vi "Scan Control Data Element.vi"(7 "Body":string, 8 "error in (no error)":errorcluster, 11 "Type/Default in":variant) -> (0 "error out":errorcluster, 3 "Type/Default out":variant)   [LabVIEW 2023, in "Request.lvclass"]
uses:
  Request.lvclass
  <vilib>/Utility/Data Type/NI_Data Type.lvlib
  <vilib>/wsapi/NI_WebServices.lvlib
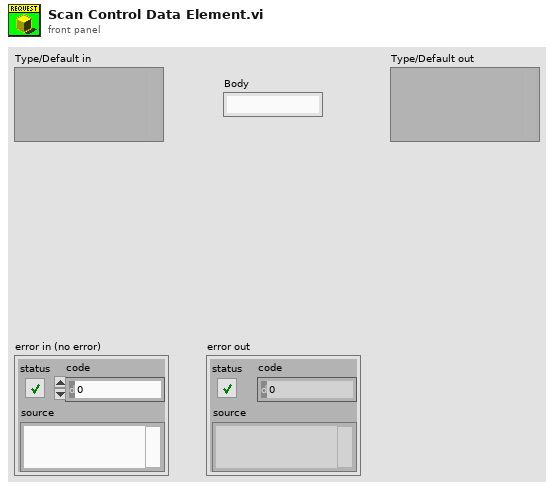
[diagram p1: front panel]
types:
  T1 = typedef "NI_Data Type.lvlib/Data Type.ctl" = enum8{"Invalid Type", "Void", "I8", "I16", "I32", "I64", "U8", "U16", "U32", "U64", "Single Float", "Double Float", "Extended Float", "Single Complex", "Double Complex", "Extended Complex", "Enum U8", "Enum U16", "Enum U32", "Enum U64", "Single Float With Unit", "Double Float With Unit", "Extended Float With Unit", "Single Complex with Unit", "Double Complex with Unit", "Extended Complex with Unit", "Boolean", "String", "Path", "Picture", "Tag", "Array", "Cluster", "Variant", "LV Variant", "Waveform", "Timestamp", "Digital Waveform", "Digital Data", "ExpressData", "Refnum", "External Data", "VI", "Poly VI", "LabVIEW Class Instance", "Fixed Point", "Set Collection", "Map Collection"}
  T2 = typedef "imagedata.ctl" = cluster{"image type":i32, "image depth":i32, "image":u8[], "mask":u8[], "colors":u32[], "Rectangle":cluster{"left":i16, "top":i16, "right":i16, "bottom":i16}}
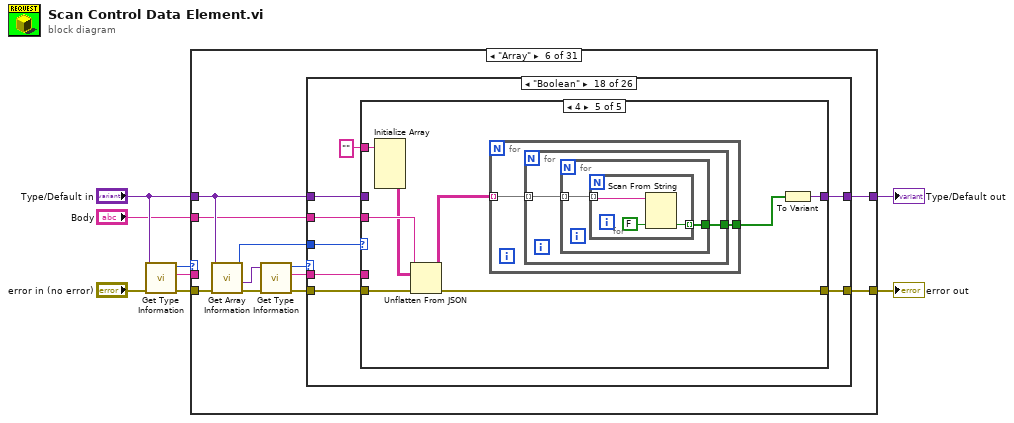
[diagram p0: block diagram]
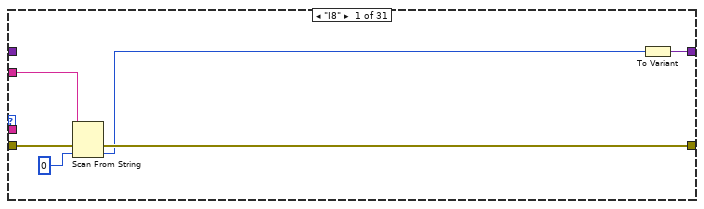
[diagram p2: hidden frame]
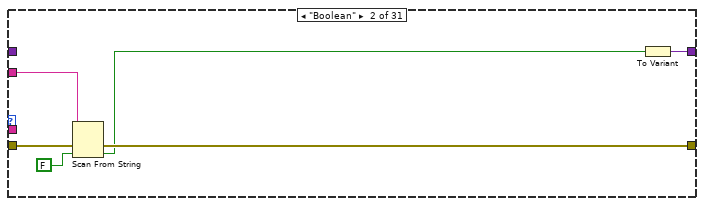
[diagram p3: hidden frame]
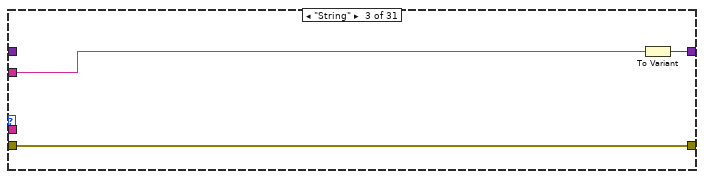
[diagram p4: hidden frame]
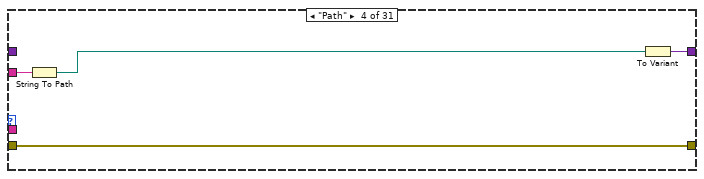
[diagram p5: hidden frame]
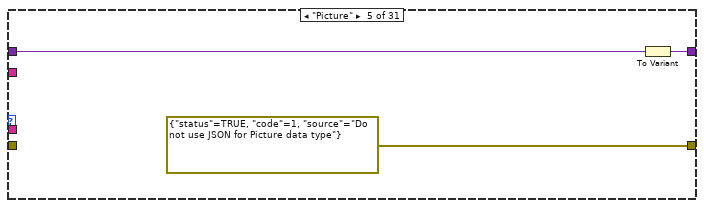
[diagram p6: hidden frame]
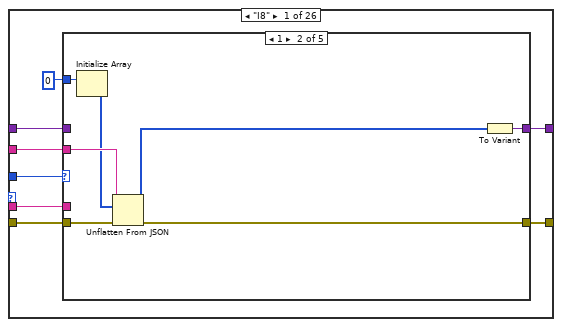
[diagram p7: hidden frame]
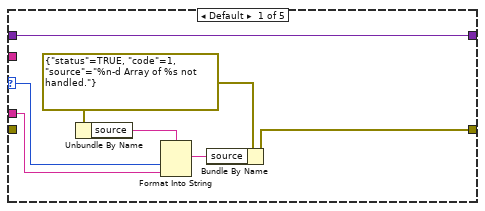
[diagram p8: hidden frame]
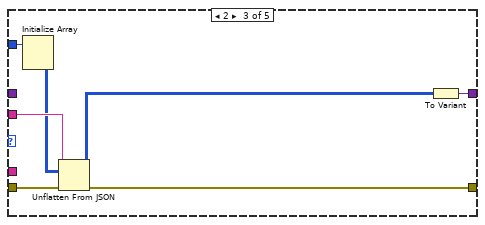
[diagram p9: hidden frame]
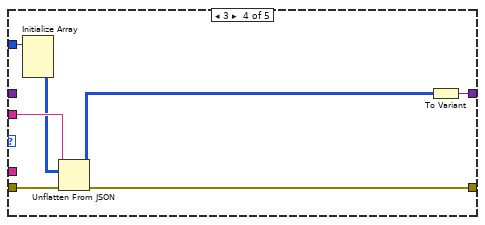
[diagram p10: hidden frame]
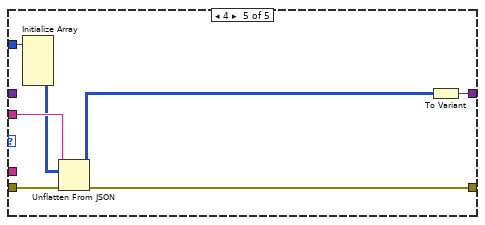
[diagram p11: hidden frame]
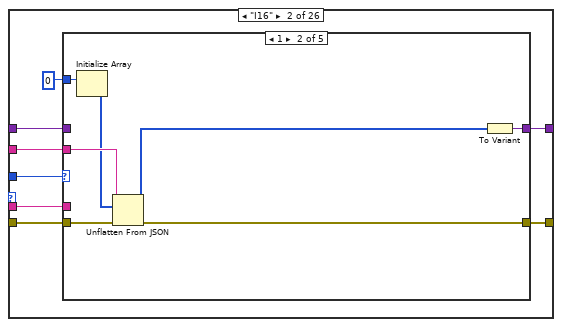
[diagram p12: hidden frame]
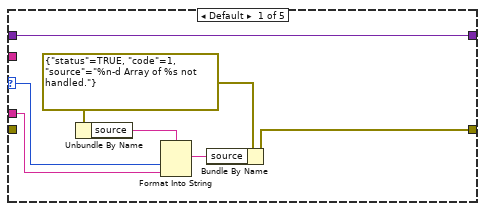
[diagram p13: hidden frame]
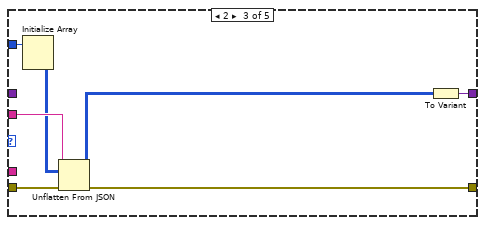
[diagram p14: hidden frame]
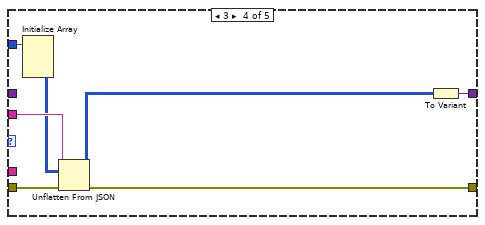
[diagram p15: hidden frame]
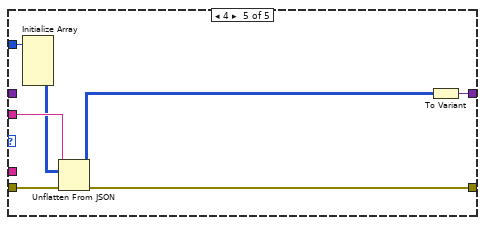
[diagram p16: hidden frame]
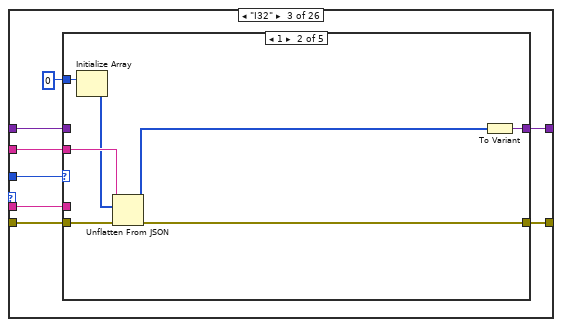
[diagram p17: hidden frame]
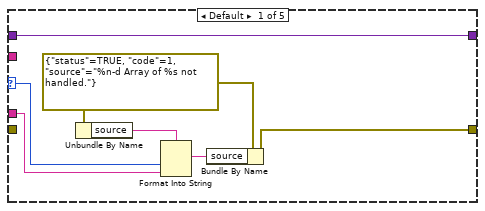
[diagram p18: hidden frame]
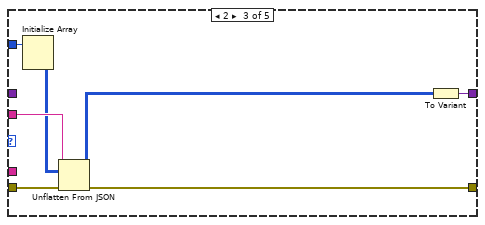
[diagram p19: hidden frame]
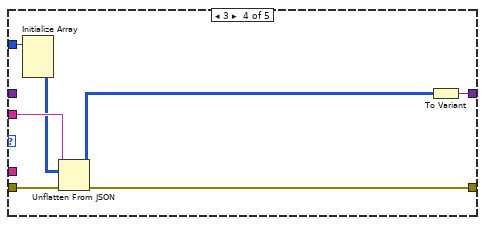
[diagram p20: hidden frame]
diagram:
  n1 = call <vilib>:"Get Type Information.vi"("error in (no error)"="error in (no error)", "variant"="Type/Default in") -> ("error out"=w7:errorcluster, "name"=w8:string, "type"=w3:T1)  [unwired: 5 in, 2 out]
  n2 = case shown="\"Array\"" w3 {
    tunnel: [w10 w16 w23 w27 w30 w41 w1308 w1330 w1336 w1342 w1348 w1354 w1360 w1366 w1372 w1378 w1384 w1390 w1396 w1402 w1408 w1414 w1420 w1426 w1432 w1438 w1450 w1458 w1466 w1474 w1480] -> w4
    tunnel: "Type/Default in" -> [_ _ _ _ w28 w39 w1308 _ _ _ _ _ _ _ _ _ _ _ _ _ _ _ _ _ _ _ w1449 w1457 w1465 w1473 w1480]
    tunnel: [w13 w19 w21 w25 errorcluster {"status"=TRUE, "code"=1, "source"="Do not use JSON for Picture data type"} ("error out") w33 w1309 w1333 w1339 w1345 w1351 w1357 w1363 w1369 w1375 w1381 w1387 w1393 w1399 w1405 w1411 w1417 w1423 w1429 w1435 w1441 w1444 w1452 w1460 w1468 w1475] -> w6
    tunnel: w7 -> [w14 w20 w21 w25 _ w40 w1312 w1334 w1340 w1346 w1352 w1358 w1364 w1370 w1376 w1382 w1388 w1394 w1400 w1406 w1412 w1418 w1424 w1430 w1436 w1442 w1448 w1456 w1464 w1472 _]
    tunnel: "Body" -> [w12 w18 w22 w26 _ w32 w1307 w1332 w1338 w1344 w1350 w1356 w1362 w1368 w1374 w1380 w1386 w1392 w1398 w1404 w1410 w1416 w1422 w1428 w1434 w1440 w1446 w1454 w1462 w1470 _]
    tunnel: w8 -> [_ _ _ _ _ _ _ _ _ _ _ _ _ _ _ _ _ _ _ _ _ _ _ _ _ _ _ _ _ _ w1477]
    frame "I8" {
      n3 = Scan From String(input string=w12, error in=w14, default 1=i8 0 ("default value 1")) -> (error out=w13:errorcluster, output 1=w9:i8)  [unwired: 2 in, 2 out]
      n4 = To Variant(anything=w9) -> (Variant=w10:variant)
    }
    frame "Boolean" {
      n5 = Scan From String(input string=w18, error in=w20, default 1=FALSE) -> (error out=w19:errorcluster, output 1=w15:bool)  [unwired: 2 in, 2 out]
      n6 = To Variant(anything=w15) -> (Variant=w16:variant)
    }
    frame "String" {
      n7 = To Variant(anything=w22) -> (Variant=w23:variant)
    }
    frame "Path" {
      n8 = String To Path(string=w26) -> (path=w24:path)
      n9 = To Variant(anything=w24) -> (Variant=w27:variant)
    }
    frame "Picture" {
      n10 = To Variant(anything=w28) -> (Variant=w30:variant)
    }
    frame "Array" {
      n11 = call <vilib>:"Get Array Information.vi"("error in (no error)"=w40, "variant"=w39) -> ("error out"=w38:errorcluster, "array element data type"=w37:variant, "number of dimensions"=w31:i32)  [unwired: 6 in, 1 out]
      n12 = call <vilib>:"Get Type Information.vi"("error in (no error)"=w38, "variant"=w37) -> ("error out"=w36:errorcluster, "name"=w34:string, "type"=w35:T1)  [unwired: 5 in, 2 out]
      n13 = case shown="\"Boolean\"" w35 {
        tunnel: [w45 w88 w131 w174 w217 w260 w303 w346 w389 w432 w475 w518 w561 w604 w647 w690 w733 w776 w847 w890 w937 w1028 w1097 w1166 w1235 w1301] -> w41
        tunnel: w39 -> [w43 w86 w129 w172 w215 w258 w301 w344 w387 w430 w473 w516 w559 w602 w645 w688 w731 w774 w845 w888 w935 w1026 w1095 w1164 w1233 w1301]
        tunnel: w36 -> [w47 w90 w133 w176 w219 w262 w305 w348 w391 w434 w477 w520 w563 w606 w649 w692 w735 w778 w849 w892 w939 w1030 w1099 w1168 w1237 _]
        tunnel: w34 -> [w42 w85 w128 w171 w214 w257 w300 w343 w386 w429 w472 w515 w558 w601 w644 w687 w730 w773 w844 w887 w934 w1025 w1094 w1163 w1232 w1303]
        tunnel: [w44 w87 w130 w173 w216 w259 w302 w345 w388 w431 w474 w517 w560 w603 w646 w689 w732 w775 w846 w889 w936 w1027 w1096 w1165 w1234 w1302] -> w33
        tunnel: w32 -> [w46 w89 w132 w175 w218 w261 w304 w347 w390 w433 w476 w519 w562 w605 w648 w691 w734 w777 w848 w891 w938 w1029 w1098 w1167 w1236 _]
        tunnel: w31 -> [w49 w92 w135 w178 w221 w264 w307 w350 w393 w436 w479 w522 w565 w608 w651 w694 w737 w780 w851 w894 w941 w1032 w1101 w1170 w1239 _]
        frame "I8" {
          n14 = case shown="1" w49 {
            selector: w49 -> [w52 _ _ _ _]
            tunnel: i8 0 -> [_ w63 w70 w77 w84]
            tunnel: w47 -> [_ w62 w69 w76 w83]
            tunnel: w46 -> [_ w61 w68 w75 w82]
            tunnel: [w56 w58 w65 w72 w79] -> w45
            tunnel: [w50 w57 w64 w71 w78] -> w44
            tunnel: w43 -> [w56 _ _ _ _]
            tunnel: w42 -> [w51 _ _ _ _]
            frame Default {
              w53 = errorcluster {"status"=TRUE, "code"=1, "source"="%n-d Array of %s not handled."} ("error out")
              n15 = Unbundle By Name(w53) -> ("source"=w54:string)
              n16 = Format Into String(format string=w54, w52, w51) -> (resulting string=w55:string)  [unwired: 2 in, 1 out]
              n17 = Bundle By Name(cluster=w53, "source"=w55) -> (w50:errorcluster)
            }
            frame 1 {
              n18 = Initialize Array(w63) -> (w60:i8[])  [unwired: 1 in]
              n19 = Unflatten From JSON(JSON string=w61, type and defaults=w60, error in (no error)=w62) -> (value=w59:i8[], error out=w57:errorcluster)  [unwired: 4 in]
              n20 = To Variant(anything=w59) -> (Variant=w58:variant)
            }
            frame 2 {
              n21 = Initialize Array(w70) -> (w67:i8[][])  [unwired: 2 in]
              n22 = Unflatten From JSON(JSON string=w68, type and defaults=w67, error in (no error)=w69) -> (value=w66:i8[][], error out=w64:errorcluster)  [unwired: 4 in]
              n23 = To Variant(anything=w66) -> (Variant=w65:variant)
            }
            frame 3 {
              n24 = Initialize Array(w77) -> (w74:i8[][][])  [unwired: 3 in]
              n25 = Unflatten From JSON(JSON string=w75, type and defaults=w74, error in (no error)=w76) -> (value=w73:i8[][][], error out=w71:errorcluster)  [unwired: 4 in]
              n26 = To Variant(anything=w73) -> (Variant=w72:variant)
            }
            frame 4 {
              n27 = Initialize Array(w84) -> (w81:i8[][][][])  [unwired: 4 in]
              n28 = Unflatten From JSON(JSON string=w82, type and defaults=w81, error in (no error)=w83) -> (value=w80:i8[][][][], error out=w78:errorcluster)  [unwired: 4 in]
              n29 = To Variant(anything=w80) -> (Variant=w79:variant)
            }
          }
        }
        frame "I16" {
          n30 = case shown="1" w92 {
            selector: w92 -> [w95 _ _ _ _]
            tunnel: i16 0 -> [_ w106 w113 w120 w127]
            tunnel: w90 -> [_ w105 w112 w119 w126]
            tunnel: w89 -> [_ w104 w111 w118 w125]
            tunnel: [w99 w101 w108 w115 w122] -> w88
            tunnel: [w93 w100 w107 w114 w121] -> w87
            tunnel: w86 -> [w99 _ _ _ _]
            tunnel: w85 -> [w94 _ _ _ _]
            frame Default {
              w96 = errorcluster {"status"=TRUE, "code"=1, "source"="%n-d Array of %s not handled."} ("error out")
              n31 = Unbundle By Name(w96) -> ("source"=w97:string)
              n32 = Format Into String(format string=w97, w95, w94) -> (resulting string=w98:string)  [unwired: 2 in, 1 out]
              n33 = Bundle By Name(cluster=w96, "source"=w98) -> (w93:errorcluster)
            }
            frame 1 {
              n34 = Initialize Array(w106) -> (w103:i16[])  [unwired: 1 in]
              n35 = Unflatten From JSON(JSON string=w104, type and defaults=w103, error in (no error)=w105) -> (value=w102:i16[], error out=w100:errorcluster)  [unwired: 4 in]
              n36 = To Variant(anything=w102) -> (Variant=w101:variant)
            }
            frame 2 {
              n37 = Initialize Array(w113) -> (w110:i16[][])  [unwired: 2 in]
              n38 = Unflatten From JSON(JSON string=w111, type and defaults=w110, error in (no error)=w112) -> (value=w109:i16[][], error out=w107:errorcluster)  [unwired: 4 in]
              n39 = To Variant(anything=w109) -> (Variant=w108:variant)
            }
            frame 3 {
              n40 = Initialize Array(w120) -> (w117:i16[][][])  [unwired: 3 in]
              n41 = Unflatten From JSON(JSON string=w118, type and defaults=w117, error in (no error)=w119) -> (value=w116:i16[][][], error out=w114:errorcluster)  [unwired: 4 in]
              n42 = To Variant(anything=w116) -> (Variant=w115:variant)
            }
            frame 4 {
              n43 = Initialize Array(w127) -> (w124:i16[][][][])  [unwired: 4 in]
              n44 = Unflatten From JSON(JSON string=w125, type and defaults=w124, error in (no error)=w126) -> (value=w123:i16[][][][], error out=w121:errorcluster)  [unwired: 4 in]
              n45 = To Variant(anything=w123) -> (Variant=w122:variant)
            }
          }
        }
        frame "I32" {
          n46 = case shown="1" w135 {
            selector: w135 -> [w138 _ _ _ _]
            tunnel: 0 -> [_ w149 w156 w163 w170]
            tunnel: w133 -> [_ w148 w155 w162 w169]
            tunnel: w132 -> [_ w147 w154 w161 w168]
            tunnel: [w142 w144 w151 w158 w165] -> w131
            tunnel: [w136 w143 w150 w157 w164] -> w130
            tunnel: w129 -> [w142 _ _ _ _]
            tunnel: w128 -> [w137 _ _ _ _]
            frame Default {
              w139 = errorcluster {"status"=TRUE, "code"=1, "source"="%n-d Array of %s not handled."} ("error out")
              n47 = Unbundle By Name(w139) -> ("source"=w140:string)
              n48 = Format Into String(format string=w140, w138, w137) -> (resulting string=w141:string)  [unwired: 2 in, 1 out]
              n49 = Bundle By Name(cluster=w139, "source"=w141) -> (w136:errorcluster)
            }
            frame 1 {
              n50 = Initialize Array(w149) -> (w146:i32[])  [unwired: 1 in]
              n51 = Unflatten From JSON(JSON string=w147, type and defaults=w146, error in (no error)=w148) -> (value=w145:i32[], error out=w143:errorcluster)  [unwired: 4 in]
              n52 = To Variant(anything=w145) -> (Variant=w144:variant)
            }
            frame 2 {
              n53 = Initialize Array(w156) -> (w153:i32[][])  [unwired: 2 in]
              n54 = Unflatten From JSON(JSON string=w154, type and defaults=w153, error in (no error)=w155) -> (value=w152:i32[][], error out=w150:errorcluster)  [unwired: 4 in]
              n55 = To Variant(anything=w152) -> (Variant=w151:variant)
            }
            frame 3 {
              n56 = Initialize Array(w163) -> (w160:i32[][][])  [unwired: 3 in]
              n57 = Unflatten From JSON(JSON string=w161, type and defaults=w160, error in (no error)=w162) -> (value=w159:i32[][][], error out=w157:errorcluster)  [unwired: 4 in]
              n58 = To Variant(anything=w159) -> (Variant=w158:variant)
            }
            frame 4 {
              n59 = Initialize Array(w170) -> (w167:i32[][][][])  [unwired: 4 in]
              n60 = Unflatten From JSON(JSON string=w168, type and defaults=w167, error in (no error)=w169) -> (value=w166:i32[][][][], error out=w164:errorcluster)  [unwired: 4 in]
              n61 = To Variant(anything=w166) -> (Variant=w165:variant)
            }
          }
        }
        frame "I64" {
          n62 = case shown="1" w178 {
            selector: w178 -> [w181 _ _ _ _]
            tunnel: i64 0 -> [_ w192 w199 w206 w213]
            tunnel: w176 -> [_ w191 w198 w205 w212]
            tunnel: w175 -> [_ w190 w197 w204 w211]
            tunnel: [w185 w187 w194 w201 w208] -> w174
            tunnel: [w179 w186 w193 w200 w207] -> w173
            tunnel: w172 -> [w185 _ _ _ _]
            tunnel: w171 -> [w180 _ _ _ _]
            frame Default {
              w182 = errorcluster {"status"=TRUE, "code"=1, "source"="%n-d Array of %s not handled."} ("error out")
              n63 = Unbundle By Name(w182) -> ("source"=w183:string)
              n64 = Format Into String(format string=w183, w181, w180) -> (resulting string=w184:string)  [unwired: 2 in, 1 out]
              n65 = Bundle By Name(cluster=w182, "source"=w184) -> (w179:errorcluster)
            }
            frame 1 {
              n66 = Initialize Array(w192) -> (w189:i64[])  [unwired: 1 in]
              n67 = Unflatten From JSON(JSON string=w190, type and defaults=w189, error in (no error)=w191) -> (value=w188:i64[], error out=w186:errorcluster)  [unwired: 4 in]
              n68 = To Variant(anything=w188) -> (Variant=w187:variant)
            }
            frame 2 {
              n69 = Initialize Array(w199) -> (w196:i64[][])  [unwired: 2 in]
              n70 = Unflatten From JSON(JSON string=w197, type and defaults=w196, error in (no error)=w198) -> (value=w195:i64[][], error out=w193:errorcluster)  [unwired: 4 in]
              n71 = To Variant(anything=w195) -> (Variant=w194:variant)
            }
            frame 3 {
              n72 = Initialize Array(w206) -> (w203:i64[][][])  [unwired: 3 in]
              n73 = Unflatten From JSON(JSON string=w204, type and defaults=w203, error in (no error)=w205) -> (value=w202:i64[][][], error out=w200:errorcluster)  [unwired: 4 in]
              n74 = To Variant(anything=w202) -> (Variant=w201:variant)
            }
            frame 4 {
              n75 = Initialize Array(w213) -> (w210:i64[][][][])  [unwired: 4 in]
              n76 = Unflatten From JSON(JSON string=w211, type and defaults=w210, error in (no error)=w212) -> (value=w209:i64[][][][], error out=w207:errorcluster)  [unwired: 4 in]
              n77 = To Variant(anything=w209) -> (Variant=w208:variant)
            }
          }
        }
        frame "U8" {
          n78 = case shown="1" w221 {
            selector: w221 -> [w224 _ _ _ _]
            tunnel: u8 0 -> [_ w235 w242 w249 w256]
            tunnel: w219 -> [_ w234 w241 w248 w255]
            tunnel: w218 -> [_ w233 w240 w247 w254]
            tunnel: [w228 w230 w237 w244 w251] -> w217
            tunnel: [w222 w229 w236 w243 w250] -> w216
            tunnel: w215 -> [w228 _ _ _ _]
            tunnel: w214 -> [w223 _ _ _ _]
            frame Default {
              w225 = errorcluster {"status"=TRUE, "code"=1, "source"="%n-d Array of %s not handled."} ("error out")
              n79 = Unbundle By Name(w225) -> ("source"=w226:string)
              n80 = Format Into String(format string=w226, w224, w223) -> (resulting string=w227:string)  [unwired: 2 in, 1 out]
              n81 = Bundle By Name(cluster=w225, "source"=w227) -> (w222:errorcluster)
            }
            frame 1 {
              n82 = Initialize Array(w235) -> (w232:u8[])  [unwired: 1 in]
              n83 = Unflatten From JSON(JSON string=w233, type and defaults=w232, error in (no error)=w234) -> (value=w231:u8[], error out=w229:errorcluster)  [unwired: 4 in]
              n84 = To Variant(anything=w231) -> (Variant=w230:variant)
            }
            frame 2 {
              n85 = Initialize Array(w242) -> (w239:u8[][])  [unwired: 2 in]
              n86 = Unflatten From JSON(JSON string=w240, type and defaults=w239, error in (no error)=w241) -> (value=w238:u8[][], error out=w236:errorcluster)  [unwired: 4 in]
              n87 = To Variant(anything=w238) -> (Variant=w237:variant)
            }
            frame 3 {
              n88 = Initialize Array(w249) -> (w246:u8[][][])  [unwired: 3 in]
              n89 = Unflatten From JSON(JSON string=w247, type and defaults=w246, error in (no error)=w248) -> (value=w245:u8[][][], error out=w243:errorcluster)  [unwired: 4 in]
              n90 = To Variant(anything=w245) -> (Variant=w244:variant)
            }
            frame 4 {
              n91 = Initialize Array(w256) -> (w253:u8[][][][])  [unwired: 4 in]
              n92 = Unflatten From JSON(JSON string=w254, type and defaults=w253, error in (no error)=w255) -> (value=w252:u8[][][][], error out=w250:errorcluster)  [unwired: 4 in]
              n93 = To Variant(anything=w252) -> (Variant=w251:variant)
            }
          }
        }
        frame "U16" {
          n94 = case shown="1" w264 {
            selector: w264 -> [w267 _ _ _ _]
            tunnel: u16 0 -> [_ w278 w285 w292 w299]
            tunnel: w262 -> [_ w277 w284 w291 w298]
            tunnel: w261 -> [_ w276 w283 w290 w297]
            tunnel: [w271 w273 w280 w287 w294] -> w260
            tunnel: [w265 w272 w279 w286 w293] -> w259
            tunnel: w258 -> [w271 _ _ _ _]
            tunnel: w257 -> [w266 _ _ _ _]
            frame Default {
              w268 = errorcluster {"status"=TRUE, "code"=1, "source"="%n-d Array of %s not handled."} ("error out")
              n95 = Unbundle By Name(w268) -> ("source"=w269:string)
              n96 = Format Into String(format string=w269, w267, w266) -> (resulting string=w270:string)  [unwired: 2 in, 1 out]
              n97 = Bundle By Name(cluster=w268, "source"=w270) -> (w265:errorcluster)
            }
            frame 1 {
              n98 = Initialize Array(w278) -> (w275:u16[])  [unwired: 1 in]
              n99 = Unflatten From JSON(JSON string=w276, type and defaults=w275, error in (no error)=w277) -> (value=w274:u16[], error out=w272:errorcluster)  [unwired: 4 in]
              n100 = To Variant(anything=w274) -> (Variant=w273:variant)
            }
            frame 2 {
              n101 = Initialize Array(w285) -> (w282:u16[][])  [unwired: 2 in]
              n102 = Unflatten From JSON(JSON string=w283, type and defaults=w282, error in (no error)=w284) -> (value=w281:u16[][], error out=w279:errorcluster)  [unwired: 4 in]
              n103 = To Variant(anything=w281) -> (Variant=w280:variant)
            }
            frame 3 {
              n104 = Initialize Array(w292) -> (w289:u16[][][])  [unwired: 3 in]
              n105 = Unflatten From JSON(JSON string=w290, type and defaults=w289, error in (no error)=w291) -> (value=w288:u16[][][], error out=w286:errorcluster)  [unwired: 4 in]
              n106 = To Variant(anything=w288) -> (Variant=w287:variant)
            }
            frame 4 {
              n107 = Initialize Array(w299) -> (w296:u16[][][][])  [unwired: 4 in]
              n108 = Unflatten From JSON(JSON string=w297, type and defaults=w296, error in (no error)=w298) -> (value=w295:u16[][][][], error out=w293:errorcluster)  [unwired: 4 in]
              n109 = To Variant(anything=w295) -> (Variant=w294:variant)
            }
          }
        }
        frame "U32" {
          n110 = case shown="1" w307 {
            selector: w307 -> [w310 _ _ _ _]
            tunnel: u32 0 -> [_ w321 w328 w335 w342]
            tunnel: w305 -> [_ w320 w327 w334 w341]
            tunnel: w304 -> [_ w319 w326 w333 w340]
            tunnel: [w314 w316 w323 w330 w337] -> w303
            tunnel: [w308 w315 w322 w329 w336] -> w302
            tunnel: w301 -> [w314 _ _ _ _]
            tunnel: w300 -> [w309 _ _ _ _]
            frame Default {
              w311 = errorcluster {"status"=TRUE, "code"=1, "source"="%n-d Array of %s not handled."} ("error out")
              n111 = Unbundle By Name(w311) -> ("source"=w312:string)
              n112 = Format Into String(format string=w312, w310, w309) -> (resulting string=w313:string)  [unwired: 2 in, 1 out]
              n113 = Bundle By Name(cluster=w311, "source"=w313) -> (w308:errorcluster)
            }
            frame 1 {
              n114 = Initialize Array(w321) -> (w318:u32[])  [unwired: 1 in]
              n115 = Unflatten From JSON(JSON string=w319, type and defaults=w318, error in (no error)=w320) -> (value=w317:u32[], error out=w315:errorcluster)  [unwired: 4 in]
              n116 = To Variant(anything=w317) -> (Variant=w316:variant)
            }
            frame 2 {
              n117 = Initialize Array(w328) -> (w325:u32[][])  [unwired: 2 in]
              n118 = Unflatten From JSON(JSON string=w326, type and defaults=w325, error in (no error)=w327) -> (value=w324:u32[][], error out=w322:errorcluster)  [unwired: 4 in]
              n119 = To Variant(anything=w324) -> (Variant=w323:variant)
            }
            frame 3 {
              n120 = Initialize Array(w335) -> (w332:u32[][][])  [unwired: 3 in]
              n121 = Unflatten From JSON(JSON string=w333, type and defaults=w332, error in (no error)=w334) -> (value=w331:u32[][][], error out=w329:errorcluster)  [unwired: 4 in]
              n122 = To Variant(anything=w331) -> (Variant=w330:variant)
            }
            frame 4 {
              n123 = Initialize Array(w342) -> (w339:u32[][][][])  [unwired: 4 in]
              n124 = Unflatten From JSON(JSON string=w340, type and defaults=w339, error in (no error)=w341) -> (value=w338:u32[][][][], error out=w336:errorcluster)  [unwired: 4 in]
              n125 = To Variant(anything=w338) -> (Variant=w337:variant)
            }
          }
        }
        frame "U64" {
          n126 = case shown="1" w350 {
            selector: w350 -> [w353 _ _ _ _]
            tunnel: u64 0 -> [_ w364 w371 w378 w385]
            tunnel: w348 -> [_ w363 w370 w377 w384]
            tunnel: w347 -> [_ w362 w369 w376 w383]
            tunnel: [w357 w359 w366 w373 w380] -> w346
            tunnel: [w351 w358 w365 w372 w379] -> w345
            tunnel: w344 -> [w357 _ _ _ _]
            tunnel: w343 -> [w352 _ _ _ _]
            frame Default {
              w354 = errorcluster {"status"=TRUE, "code"=1, "source"="%n-d Array of %s not handled."} ("error out")
              n127 = Unbundle By Name(w354) -> ("source"=w355:string)
              n128 = Format Into String(format string=w355, w353, w352) -> (resulting string=w356:string)  [unwired: 2 in, 1 out]
              n129 = Bundle By Name(cluster=w354, "source"=w356) -> (w351:errorcluster)
            }
            frame 1 {
              n130 = Initialize Array(w364) -> (w361:u64[])  [unwired: 1 in]
              n131 = Unflatten From JSON(JSON string=w362, type and defaults=w361, error in (no error)=w363) -> (value=w360:u64[], error out=w358:errorcluster)  [unwired: 4 in]
              n132 = To Variant(anything=w360) -> (Variant=w359:variant)
            }
            frame 2 {
              n133 = Initialize Array(w371) -> (w368:u64[][])  [unwired: 2 in]
              n134 = Unflatten From JSON(JSON string=w369, type and defaults=w368, error in (no error)=w370) -> (value=w367:u64[][], error out=w365:errorcluster)  [unwired: 4 in]
              n135 = To Variant(anything=w367) -> (Variant=w366:variant)
            }
            frame 3 {
              n136 = Initialize Array(w378) -> (w375:u64[][][])  [unwired: 3 in]
              n137 = Unflatten From JSON(JSON string=w376, type and defaults=w375, error in (no error)=w377) -> (value=w374:u64[][][], error out=w372:errorcluster)  [unwired: 4 in]
              n138 = To Variant(anything=w374) -> (Variant=w373:variant)
            }
            frame 4 {
              n139 = Initialize Array(w385) -> (w382:u64[][][][])  [unwired: 4 in]
              n140 = Unflatten From JSON(JSON string=w383, type and defaults=w382, error in (no error)=w384) -> (value=w381:u64[][][][], error out=w379:errorcluster)  [unwired: 4 in]
              n141 = To Variant(anything=w381) -> (Variant=w380:variant)
            }
          }
        }
        frame "Single Float" {
          n142 = case shown="1" w393 {
            selector: w393 -> [w396 _ _ _ _]
            tunnel: sgl 0.0 -> [_ w407 w414 w421 w428]
            tunnel: w391 -> [_ w406 w413 w420 w427]
            tunnel: w390 -> [_ w405 w412 w419 w426]
            tunnel: [w400 w402 w409 w416 w423] -> w389
            tunnel: [w394 w401 w408 w415 w422] -> w388
            tunnel: w387 -> [w400 _ _ _ _]
            tunnel: w386 -> [w395 _ _ _ _]
            frame Default {
              w397 = errorcluster {"status"=TRUE, "code"=1, "source"="%n-d Array of %s not handled."} ("error out")
              n143 = Unbundle By Name(w397) -> ("source"=w398:string)
              n144 = Format Into String(format string=w398, w396, w395) -> (resulting string=w399:string)  [unwired: 2 in, 1 out]
              n145 = Bundle By Name(cluster=w397, "source"=w399) -> (w394:errorcluster)
            }
            frame 1 {
              n146 = Initialize Array(w407) -> (w404:sgl[])  [unwired: 1 in]
              n147 = Unflatten From JSON(JSON string=w405, type and defaults=w404, error in (no error)=w406) -> (value=w403:sgl[], error out=w401:errorcluster)  [unwired: 4 in]
              n148 = To Variant(anything=w403) -> (Variant=w402:variant)
            }
            frame 2 {
              n149 = Initialize Array(w414) -> (w411:sgl[][])  [unwired: 2 in]
              n150 = Unflatten From JSON(JSON string=w412, type and defaults=w411, error in (no error)=w413) -> (value=w410:sgl[][], error out=w408:errorcluster)  [unwired: 4 in]
              n151 = To Variant(anything=w410) -> (Variant=w409:variant)
            }
            frame 3 {
              n152 = Initialize Array(w421) -> (w418:sgl[][][])  [unwired: 3 in]
              n153 = Unflatten From JSON(JSON string=w419, type and defaults=w418, error in (no error)=w420) -> (value=w417:sgl[][][], error out=w415:errorcluster)  [unwired: 4 in]
              n154 = To Variant(anything=w417) -> (Variant=w416:variant)
            }
            frame 4 {
              n155 = Initialize Array(w428) -> (w425:sgl[][][][])  [unwired: 4 in]
              n156 = Unflatten From JSON(JSON string=w426, type and defaults=w425, error in (no error)=w427) -> (value=w424:sgl[][][][], error out=w422:errorcluster)  [unwired: 4 in]
              n157 = To Variant(anything=w424) -> (Variant=w423:variant)
            }
          }
        }
        frame "Single Float With Unit" {
          n158 = case shown="1" w436 {
            selector: w436 -> [w439 _ _ _ _]
            tunnel: sgl 0.0 -> [_ w450 w457 w464 w471]
            tunnel: w434 -> [_ w449 w456 w463 w470]
            tunnel: w433 -> [_ w448 w455 w462 w469]
            tunnel: [w443 w445 w452 w459 w466] -> w432
            tunnel: [w437 w444 w451 w458 w465] -> w431
            tunnel: w430 -> [w443 _ _ _ _]
            tunnel: w429 -> [w438 _ _ _ _]
            frame Default {
              w440 = errorcluster {"status"=TRUE, "code"=1, "source"="%n-d Array of %s not handled."} ("error out")
              n159 = Unbundle By Name(w440) -> ("source"=w441:string)
              n160 = Format Into String(format string=w441, w439, w438) -> (resulting string=w442:string)  [unwired: 2 in, 1 out]
              n161 = Bundle By Name(cluster=w440, "source"=w442) -> (w437:errorcluster)
            }
            frame 1 {
              n162 = Initialize Array(w450) -> (w447:sgl[])  [unwired: 1 in]
              n163 = Unflatten From JSON(JSON string=w448, type and defaults=w447, error in (no error)=w449) -> (value=w446:sgl[], error out=w444:errorcluster)  [unwired: 4 in]
              n164 = To Variant(anything=w446) -> (Variant=w445:variant)
            }
            frame 2 {
              n165 = Initialize Array(w457) -> (w454:sgl[][])  [unwired: 2 in]
              n166 = Unflatten From JSON(JSON string=w455, type and defaults=w454, error in (no error)=w456) -> (value=w453:sgl[][], error out=w451:errorcluster)  [unwired: 4 in]
              n167 = To Variant(anything=w453) -> (Variant=w452:variant)
            }
            frame 3 {
              n168 = Initialize Array(w464) -> (w461:sgl[][][])  [unwired: 3 in]
              n169 = Unflatten From JSON(JSON string=w462, type and defaults=w461, error in (no error)=w463) -> (value=w460:sgl[][][], error out=w458:errorcluster)  [unwired: 4 in]
              n170 = To Variant(anything=w460) -> (Variant=w459:variant)
            }
            frame 4 {
              n171 = Initialize Array(w471) -> (w468:sgl[][][][])  [unwired: 4 in]
              n172 = Unflatten From JSON(JSON string=w469, type and defaults=w468, error in (no error)=w470) -> (value=w467:sgl[][][][], error out=w465:errorcluster)  [unwired: 4 in]
              n173 = To Variant(anything=w467) -> (Variant=w466:variant)
            }
          }
        }
        frame "Double Float" {
          n174 = case shown="1" w479 {
            selector: w479 -> [w482 _ _ _ _]
            tunnel: 0.0 -> [_ w493 w500 w507 w514]
            tunnel: w477 -> [_ w492 w499 w506 w513]
            tunnel: w476 -> [_ w491 w498 w505 w512]
            tunnel: [w486 w488 w495 w502 w509] -> w475
            tunnel: [w480 w487 w494 w501 w508] -> w474
            tunnel: w473 -> [w486 _ _ _ _]
            tunnel: w472 -> [w481 _ _ _ _]
            frame Default {
              w483 = errorcluster {"status"=TRUE, "code"=1, "source"="%n-d Array of %s not handled."} ("error out")
              n175 = Unbundle By Name(w483) -> ("source"=w484:string)
              n176 = Format Into String(format string=w484, w482, w481) -> (resulting string=w485:string)  [unwired: 2 in, 1 out]
              n177 = Bundle By Name(cluster=w483, "source"=w485) -> (w480:errorcluster)
            }
            frame 1 {
              n178 = Initialize Array(w493) -> (w490:dbl[])  [unwired: 1 in]
              n179 = Unflatten From JSON(JSON string=w491, type and defaults=w490, error in (no error)=w492) -> (value=w489:dbl[], error out=w487:errorcluster)  [unwired: 4 in]
              n180 = To Variant(anything=w489) -> (Variant=w488:variant)
            }
            frame 2 {
              n181 = Initialize Array(w500) -> (w497:dbl[][])  [unwired: 2 in]
              n182 = Unflatten From JSON(JSON string=w498, type and defaults=w497, error in (no error)=w499) -> (value=w496:dbl[][], error out=w494:errorcluster)  [unwired: 4 in]
              n183 = To Variant(anything=w496) -> (Variant=w495:variant)
            }
            frame 3 {
              n184 = Initialize Array(w507) -> (w504:dbl[][][])  [unwired: 3 in]
              n185 = Unflatten From JSON(JSON string=w505, type and defaults=w504, error in (no error)=w506) -> (value=w503:dbl[][][], error out=w501:errorcluster)  [unwired: 4 in]
              n186 = To Variant(anything=w503) -> (Variant=w502:variant)
            }
            frame 4 {
              n187 = Initialize Array(w514) -> (w511:dbl[][][][])  [unwired: 4 in]
              n188 = Unflatten From JSON(JSON string=w512, type and defaults=w511, error in (no error)=w513) -> (value=w510:dbl[][][][], error out=w508:errorcluster)  [unwired: 4 in]
              n189 = To Variant(anything=w510) -> (Variant=w509:variant)
            }
          }
        }
        frame "Double Float With Unit" {
          n190 = case shown="1" w522 {
            selector: w522 -> [w525 _ _ _ _]
            tunnel: 0.0 -> [_ w536 w543 w550 w557]
            tunnel: w520 -> [_ w535 w542 w549 w556]
            tunnel: w519 -> [_ w534 w541 w548 w555]
            tunnel: [w529 w531 w538 w545 w552] -> w518
            tunnel: [w523 w530 w537 w544 w551] -> w517
            tunnel: w516 -> [w529 _ _ _ _]
            tunnel: w515 -> [w524 _ _ _ _]
            frame Default {
              w526 = errorcluster {"status"=TRUE, "code"=1, "source"="%n-d Array of %s not handled."} ("error out")
              n191 = Unbundle By Name(w526) -> ("source"=w527:string)
              n192 = Format Into String(format string=w527, w525, w524) -> (resulting string=w528:string)  [unwired: 2 in, 1 out]
              n193 = Bundle By Name(cluster=w526, "source"=w528) -> (w523:errorcluster)
            }
            frame 1 {
              n194 = Initialize Array(w536) -> (w533:dbl[])  [unwired: 1 in]
              n195 = Unflatten From JSON(JSON string=w534, type and defaults=w533, error in (no error)=w535) -> (value=w532:dbl[], error out=w530:errorcluster)  [unwired: 4 in]
              n196 = To Variant(anything=w532) -> (Variant=w531:variant)
            }
            frame 2 {
              n197 = Initialize Array(w543) -> (w540:dbl[][])  [unwired: 2 in]
              n198 = Unflatten From JSON(JSON string=w541, type and defaults=w540, error in (no error)=w542) -> (value=w539:dbl[][], error out=w537:errorcluster)  [unwired: 4 in]
              n199 = To Variant(anything=w539) -> (Variant=w538:variant)
            }
            frame 3 {
              n200 = Initialize Array(w550) -> (w547:dbl[][][])  [unwired: 3 in]
              n201 = Unflatten From JSON(JSON string=w548, type and defaults=w547, error in (no error)=w549) -> (value=w546:dbl[][][], error out=w544:errorcluster)  [unwired: 4 in]
              n202 = To Variant(anything=w546) -> (Variant=w545:variant)
            }
            frame 4 {
              n203 = Initialize Array(w557) -> (w554:dbl[][][][])  [unwired: 4 in]
              n204 = Unflatten From JSON(JSON string=w555, type and defaults=w554, error in (no error)=w556) -> (value=w553:dbl[][][][], error out=w551:errorcluster)  [unwired: 4 in]
              n205 = To Variant(anything=w553) -> (Variant=w552:variant)
            }
          }
        }
        frame "Extended Float" {
          n206 = case shown="1" w565 {
            selector: w565 -> [w568 _ _ _ _]
            tunnel: ext 0.0 -> [_ w579 w586 w593 w600]
            tunnel: w563 -> [_ w578 w585 w592 w599]
            tunnel: w562 -> [_ w577 w584 w591 w598]
            tunnel: [w572 w574 w581 w588 w595] -> w561
            tunnel: [w566 w573 w580 w587 w594] -> w560
            tunnel: w559 -> [w572 _ _ _ _]
            tunnel: w558 -> [w567 _ _ _ _]
            frame Default {
              w569 = errorcluster {"status"=TRUE, "code"=1, "source"="%n-d Array of %s not handled."} ("error out")
              n207 = Unbundle By Name(w569) -> ("source"=w570:string)
              n208 = Format Into String(format string=w570, w568, w567) -> (resulting string=w571:string)  [unwired: 2 in, 1 out]
              n209 = Bundle By Name(cluster=w569, "source"=w571) -> (w566:errorcluster)
            }
            frame 1 {
              n210 = Initialize Array(w579) -> (w576:ext[])  [unwired: 1 in]
              n211 = Unflatten From JSON(JSON string=w577, type and defaults=w576, error in (no error)=w578) -> (value=w575:ext[], error out=w573:errorcluster)  [unwired: 4 in]
              n212 = To Variant(anything=w575) -> (Variant=w574:variant)
            }
            frame 2 {
              n213 = Initialize Array(w586) -> (w583:ext[][])  [unwired: 2 in]
              n214 = Unflatten From JSON(JSON string=w584, type and defaults=w583, error in (no error)=w585) -> (value=w582:ext[][], error out=w580:errorcluster)  [unwired: 4 in]
              n215 = To Variant(anything=w582) -> (Variant=w581:variant)
            }
            frame 3 {
              n216 = Initialize Array(w593) -> (w590:ext[][][])  [unwired: 3 in]
              n217 = Unflatten From JSON(JSON string=w591, type and defaults=w590, error in (no error)=w592) -> (value=w589:ext[][][], error out=w587:errorcluster)  [unwired: 4 in]
              n218 = To Variant(anything=w589) -> (Variant=w588:variant)
            }
            frame 4 {
              n219 = Initialize Array(w600) -> (w597:ext[][][][])  [unwired: 4 in]
              n220 = Unflatten From JSON(JSON string=w598, type and defaults=w597, error in (no error)=w599) -> (value=w596:ext[][][][], error out=w594:errorcluster)  [unwired: 4 in]
              n221 = To Variant(anything=w596) -> (Variant=w595:variant)
            }
          }
        }
        frame "Extended Float With Unit" {
          n222 = case shown="1" w608 {
            selector: w608 -> [w611 _ _ _ _]
            tunnel: ext 0.0 -> [_ w622 w629 w636 w643]
            tunnel: w606 -> [_ w621 w628 w635 w642]
            tunnel: w605 -> [_ w620 w627 w634 w641]
            tunnel: [w615 w617 w624 w631 w638] -> w604
            tunnel: [w609 w616 w623 w630 w637] -> w603
            tunnel: w602 -> [w615 _ _ _ _]
            tunnel: w601 -> [w610 _ _ _ _]
            frame Default {
              w612 = errorcluster {"status"=TRUE, "code"=1, "source"="%n-d Array of %s not handled."} ("error out")
              n223 = Unbundle By Name(w612) -> ("source"=w613:string)
              n224 = Format Into String(format string=w613, w611, w610) -> (resulting string=w614:string)  [unwired: 2 in, 1 out]
              n225 = Bundle By Name(cluster=w612, "source"=w614) -> (w609:errorcluster)
            }
            frame 1 {
              n226 = Initialize Array(w622) -> (w619:ext[])  [unwired: 1 in]
              n227 = Unflatten From JSON(JSON string=w620, type and defaults=w619, error in (no error)=w621) -> (value=w618:ext[], error out=w616:errorcluster)  [unwired: 4 in]
              n228 = To Variant(anything=w618) -> (Variant=w617:variant)
            }
            frame 2 {
              n229 = Initialize Array(w629) -> (w626:ext[][])  [unwired: 2 in]
              n230 = Unflatten From JSON(JSON string=w627, type and defaults=w626, error in (no error)=w628) -> (value=w625:ext[][], error out=w623:errorcluster)  [unwired: 4 in]
              n231 = To Variant(anything=w625) -> (Variant=w624:variant)
            }
            frame 3 {
              n232 = Initialize Array(w636) -> (w633:ext[][][])  [unwired: 3 in]
              n233 = Unflatten From JSON(JSON string=w634, type and defaults=w633, error in (no error)=w635) -> (value=w632:ext[][][], error out=w630:errorcluster)  [unwired: 4 in]
              n234 = To Variant(anything=w632) -> (Variant=w631:variant)
            }
            frame 4 {
              n235 = Initialize Array(w643) -> (w640:ext[][][][])  [unwired: 4 in]
              n236 = Unflatten From JSON(JSON string=w641, type and defaults=w640, error in (no error)=w642) -> (value=w639:ext[][][][], error out=w637:errorcluster)  [unwired: 4 in]
              n237 = To Variant(anything=w639) -> (Variant=w638:variant)
            }
          }
        }
        frame "Single Complex with Unit" {
          n238 = case shown="1" w651 {
            selector: w651 -> [w654 _ _ _ _]
            tunnel: ext 0.0 -> [_ w665 w672 w679 w686]
            tunnel: w649 -> [_ w664 w671 w678 w685]
            tunnel: w648 -> [_ w663 w670 w677 w684]
            tunnel: [w658 w660 w667 w674 w681] -> w647
            tunnel: [w652 w659 w666 w673 w680] -> w646
            tunnel: w645 -> [w658 _ _ _ _]
            tunnel: w644 -> [w653 _ _ _ _]
            frame Default {
              w655 = errorcluster {"status"=TRUE, "code"=1, "source"="%n-d Array of %s not handled."} ("error out")
              n239 = Unbundle By Name(w655) -> ("source"=w656:string)
              n240 = Format Into String(format string=w656, w654, w653) -> (resulting string=w657:string)  [unwired: 2 in, 1 out]
              n241 = Bundle By Name(cluster=w655, "source"=w657) -> (w652:errorcluster)
            }
            frame 1 {
              n242 = Initialize Array(w665) -> (w662:ext[])  [unwired: 1 in]
              n243 = Unflatten From JSON(JSON string=w663, type and defaults=w662, error in (no error)=w664) -> (value=w661:ext[], error out=w659:errorcluster)  [unwired: 4 in]
              n244 = To Variant(anything=w661) -> (Variant=w660:variant)
            }
            frame 2 {
              n245 = Initialize Array(w672) -> (w669:ext[][])  [unwired: 2 in]
              n246 = Unflatten From JSON(JSON string=w670, type and defaults=w669, error in (no error)=w671) -> (value=w668:ext[][], error out=w666:errorcluster)  [unwired: 4 in]
              n247 = To Variant(anything=w668) -> (Variant=w667:variant)
            }
            frame 3 {
              n248 = Initialize Array(w679) -> (w676:ext[][][])  [unwired: 3 in]
              n249 = Unflatten From JSON(JSON string=w677, type and defaults=w676, error in (no error)=w678) -> (value=w675:ext[][][], error out=w673:errorcluster)  [unwired: 4 in]
              n250 = To Variant(anything=w675) -> (Variant=w674:variant)
            }
            frame 4 {
              n251 = Initialize Array(w686) -> (w683:ext[][][][])  [unwired: 4 in]
              n252 = Unflatten From JSON(JSON string=w684, type and defaults=w683, error in (no error)=w685) -> (value=w682:ext[][][][], error out=w680:errorcluster)  [unwired: 4 in]
              n253 = To Variant(anything=w682) -> (Variant=w681:variant)
            }
          }
        }
        frame "Double Complex with Unit" {
          n254 = case shown="1" w694 {
            selector: w694 -> [w697 _ _ _ _]
            tunnel: ext 0.0 -> [_ w708 w715 w722 w729]
            tunnel: w692 -> [_ w707 w714 w721 w728]
            tunnel: w691 -> [_ w706 w713 w720 w727]
            tunnel: [w701 w703 w710 w717 w724] -> w690
            tunnel: [w695 w702 w709 w716 w723] -> w689
            tunnel: w688 -> [w701 _ _ _ _]
            tunnel: w687 -> [w696 _ _ _ _]
            frame Default {
              w698 = errorcluster {"status"=TRUE, "code"=1, "source"="%n-d Array of %s not handled."} ("error out")
              n255 = Unbundle By Name(w698) -> ("source"=w699:string)
              n256 = Format Into String(format string=w699, w697, w696) -> (resulting string=w700:string)  [unwired: 2 in, 1 out]
              n257 = Bundle By Name(cluster=w698, "source"=w700) -> (w695:errorcluster)
            }
            frame 1 {
              n258 = Initialize Array(w708) -> (w705:ext[])  [unwired: 1 in]
              n259 = Unflatten From JSON(JSON string=w706, type and defaults=w705, error in (no error)=w707) -> (value=w704:ext[], error out=w702:errorcluster)  [unwired: 4 in]
              n260 = To Variant(anything=w704) -> (Variant=w703:variant)
            }
            frame 2 {
              n261 = Initialize Array(w715) -> (w712:ext[][])  [unwired: 2 in]
              n262 = Unflatten From JSON(JSON string=w713, type and defaults=w712, error in (no error)=w714) -> (value=w711:ext[][], error out=w709:errorcluster)  [unwired: 4 in]
              n263 = To Variant(anything=w711) -> (Variant=w710:variant)
            }
            frame 3 {
              n264 = Initialize Array(w722) -> (w719:ext[][][])  [unwired: 3 in]
              n265 = Unflatten From JSON(JSON string=w720, type and defaults=w719, error in (no error)=w721) -> (value=w718:ext[][][], error out=w716:errorcluster)  [unwired: 4 in]
              n266 = To Variant(anything=w718) -> (Variant=w717:variant)
            }
            frame 4 {
              n267 = Initialize Array(w729) -> (w726:ext[][][][])  [unwired: 4 in]
              n268 = Unflatten From JSON(JSON string=w727, type and defaults=w726, error in (no error)=w728) -> (value=w725:ext[][][][], error out=w723:errorcluster)  [unwired: 4 in]
              n269 = To Variant(anything=w725) -> (Variant=w724:variant)
            }
          }
        }
        frame "Extended Complex with Unit" {
          n270 = case shown="1" w737 {
            selector: w737 -> [w740 _ _ _ _]
            tunnel: ext 0.0 -> [_ w751 w758 w765 w772]
            tunnel: w735 -> [_ w750 w757 w764 w771]
            tunnel: w734 -> [_ w749 w756 w763 w770]
            tunnel: [w744 w746 w753 w760 w767] -> w733
            tunnel: [w738 w745 w752 w759 w766] -> w732
            tunnel: w731 -> [w744 _ _ _ _]
            tunnel: w730 -> [w739 _ _ _ _]
            frame Default {
              w741 = errorcluster {"status"=TRUE, "code"=1, "source"="%n-d Array of %s not handled."} ("error out")
              n271 = Unbundle By Name(w741) -> ("source"=w742:string)
              n272 = Format Into String(format string=w742, w740, w739) -> (resulting string=w743:string)  [unwired: 2 in, 1 out]
              n273 = Bundle By Name(cluster=w741, "source"=w743) -> (w738:errorcluster)
            }
            frame 1 {
              n274 = Initialize Array(w751) -> (w748:ext[])  [unwired: 1 in]
              n275 = Unflatten From JSON(JSON string=w749, type and defaults=w748, error in (no error)=w750) -> (value=w747:ext[], error out=w745:errorcluster)  [unwired: 4 in]
              n276 = To Variant(anything=w747) -> (Variant=w746:variant)
            }
            frame 2 {
              n277 = Initialize Array(w758) -> (w755:ext[][])  [unwired: 2 in]
              n278 = Unflatten From JSON(JSON string=w756, type and defaults=w755, error in (no error)=w757) -> (value=w754:ext[][], error out=w752:errorcluster)  [unwired: 4 in]
              n279 = To Variant(anything=w754) -> (Variant=w753:variant)
            }
            frame 3 {
              n280 = Initialize Array(w765) -> (w762:ext[][][])  [unwired: 3 in]
              n281 = Unflatten From JSON(JSON string=w763, type and defaults=w762, error in (no error)=w764) -> (value=w761:ext[][][], error out=w759:errorcluster)  [unwired: 4 in]
              n282 = To Variant(anything=w761) -> (Variant=w760:variant)
            }
            frame 4 {
              n283 = Initialize Array(w772) -> (w769:ext[][][][])  [unwired: 4 in]
              n284 = Unflatten From JSON(JSON string=w770, type and defaults=w769, error in (no error)=w771) -> (value=w768:ext[][][][], error out=w766:errorcluster)  [unwired: 4 in]
              n285 = To Variant(anything=w768) -> (Variant=w767:variant)
            }
          }
        }
        frame "Boolean" {
          n286 = case shown="4" w780 {
            selector: w780 -> [w783 _ _ _ _]
            tunnel: "" -> [_ w795 w806 w819 w834]
            tunnel: w778 -> [_ w794 w805 w818 w833]
            tunnel: w777 -> [_ w793 w804 w817 w832]
            tunnel: [w787 w791 w802 w815 w830] -> w776
            tunnel: [w781 w790 w801 w814 w829] -> w775
            tunnel: w774 -> [w787 _ _ _ _]
            tunnel: w773 -> [w782 _ _ _ _]
            frame Default {
              w784 = errorcluster {"status"=TRUE, "code"=1, "source"="%n-d Array of %s not handled."} ("error out")
              n287 = Unbundle By Name(w784) -> ("source"=w785:string)
              n288 = Format Into String(format string=w785, w783, w782) -> (resulting string=w786:string)  [unwired: 2 in, 1 out]
              n289 = Bundle By Name(cluster=w784, "source"=w786) -> (w781:errorcluster)
            }
            frame 1 {
              n290 = Initialize Array(w795) -> (w792:string[])  [unwired: 1 in]
              n291 = Unflatten From JSON(JSON string=w793, type and defaults=w792, error in (no error)=w794) -> (value=w789:string[], error out=w790:errorcluster)  [unwired: 4 in]
              n292 = for {
                tunnel: w789 -> [w798] mode=indexing
                tunnel: [w796] -> w788 mode=indexing
                n293 = Scan From String(input string=w798, default 1=FALSE) -> (output 1=w796:bool)  [unwired: 3 in, 3 out]
              }
              n294 = To Variant(anything=w788) -> (Variant=w791:variant)
            }
            frame 2 {
              n295 = Initialize Array(w806) -> (w803:string[][])  [unwired: 2 in]
              n296 = Unflatten From JSON(JSON string=w804, type and defaults=w803, error in (no error)=w805) -> (value=w800:string[][], error out=w801:errorcluster)  [unwired: 4 in]
              n297 = for {
                tunnel: w800 -> [w808] mode=indexing
                tunnel: [w807] -> w799
                n298 = for {
                  tunnel: w808 -> [w811] mode=indexing
                  tunnel: [w809] -> w807 mode=indexing
                  n299 = Scan From String(input string=w811, default 1=FALSE) -> (output 1=w809:bool)  [unwired: 3 in, 3 out]
                }
              }
              n300 = To Variant(anything=w799) -> (Variant=w802:variant)
            }
            frame 3 {
              n301 = Initialize Array(w819) -> (w816:string[][][])  [unwired: 3 in]
              n302 = Unflatten From JSON(JSON string=w817, type and defaults=w816, error in (no error)=w818) -> (value=w813:string[][][], error out=w814:errorcluster)  [unwired: 4 in]
              n303 = for {
                tunnel: w813 -> [w821] mode=indexing
                tunnel: [w820] -> w812
                n304 = for {
                  tunnel: w821 -> [w823] mode=indexing
                  tunnel: [w822] -> w820
                  n305 = for {
                    tunnel: w823 -> [w826] mode=indexing
                    tunnel: [w824] -> w822 mode=indexing
                    n306 = Scan From String(input string=w826, default 1=FALSE) -> (output 1=w824:bool)  [unwired: 3 in, 3 out]
                  }
                }
              }
              n307 = To Variant(anything=w812) -> (Variant=w815:variant)
            }
            frame 4 {
              n308 = Initialize Array(w834) -> (w831:string[][][][])  [unwired: 4 in]
              n309 = Unflatten From JSON(JSON string=w832, type and defaults=w831, error in (no error)=w833) -> (value=w828:string[][][][], error out=w829:errorcluster)  [unwired: 4 in]
              n310 = for {
                tunnel: w828 -> [w836] mode=indexing
                tunnel: [w835] -> w827
                n311 = for {
                  tunnel: w836 -> [w838] mode=indexing
                  tunnel: [w837] -> w835
                  n312 = for {
                    tunnel: w838 -> [w840] mode=indexing
                    tunnel: [w839] -> w837
                    n313 = for {
                      tunnel: w840 -> [w843] mode=indexing
                      tunnel: [w841] -> w839 mode=indexing
                      n314 = Scan From String(input string=w843, default 1=FALSE) -> (output 1=w841:bool)  [unwired: 3 in, 3 out]
                    }
                  }
                }
              }
              n315 = To Variant(anything=w827) -> (Variant=w830:variant)
            }
          }
        }
        frame "String" {
          n316 = case shown="1" w851 {
            selector: w851 -> [w854 _ _ _ _]
            tunnel: "" -> [_ w865 w872 w879 w886]
            tunnel: w849 -> [_ w864 w871 w878 w885]
            tunnel: w848 -> [_ w863 w870 w877 w884]
            tunnel: [w858 w860 w867 w874 w881] -> w847
            tunnel: [w852 w859 w866 w873 w880] -> w846
            tunnel: w845 -> [w858 _ _ _ _]
            tunnel: w844 -> [w853 _ _ _ _]
            frame Default {
              w855 = errorcluster {"status"=TRUE, "code"=1, "source"="%n-d Array of %s not handled."} ("error out")
              n317 = Unbundle By Name(w855) -> ("source"=w856:string)
              n318 = Format Into String(format string=w856, w854, w853) -> (resulting string=w857:string)  [unwired: 2 in, 1 out]
              n319 = Bundle By Name(cluster=w855, "source"=w857) -> (w852:errorcluster)
            }
            frame 1 {
              n320 = Initialize Array(w865) -> (w862:string[])  [unwired: 1 in]
              n321 = Unflatten From JSON(JSON string=w863, type and defaults=w862, error in (no error)=w864) -> (value=w861:string[], error out=w859:errorcluster)  [unwired: 4 in]
              n322 = To Variant(anything=w861) -> (Variant=w860:variant)
            }
            frame 2 {
              n323 = Initialize Array(w872) -> (w869:string[][])  [unwired: 2 in]
              n324 = Unflatten From JSON(JSON string=w870, type and defaults=w869, error in (no error)=w871) -> (value=w868:string[][], error out=w866:errorcluster)  [unwired: 4 in]
              n325 = To Variant(anything=w868) -> (Variant=w867:variant)
            }
            frame 3 {
              n326 = Initialize Array(w879) -> (w876:string[][][])  [unwired: 3 in]
              n327 = Unflatten From JSON(JSON string=w877, type and defaults=w876, error in (no error)=w878) -> (value=w875:string[][][], error out=w873:errorcluster)  [unwired: 4 in]
              n328 = To Variant(anything=w875) -> (Variant=w874:variant)
            }
            frame 4 {
              n329 = Initialize Array(w886) -> (w883:string[][][][])  [unwired: 4 in]
              n330 = Unflatten From JSON(JSON string=w884, type and defaults=w883, error in (no error)=w885) -> (value=w882:string[][][][], error out=w880:errorcluster)  [unwired: 4 in]
              n331 = To Variant(anything=w882) -> (Variant=w881:variant)
            }
          }
        }
        frame "Path" {
          n332 = case shown="1" w894 {
            selector: w894 -> [w897 _ _ _ _]
            tunnel: "" -> [_ w909 w917 w925 w933]
            tunnel: w892 -> [_ w908 w916 w924 w932]
            tunnel: w891 -> [_ w907 w915 w923 w931]
            tunnel: [w901 w904 w912 w920 w928] -> w890
            tunnel: [w895 w903 w911 w919 w927] -> w889
            tunnel: w888 -> [w901 _ _ _ _]
            tunnel: w887 -> [w896 _ _ _ _]
            frame Default {
              w898 = errorcluster {"status"=TRUE, "code"=1, "source"="%n-d Array of %s not handled."} ("error out")
              n333 = Unbundle By Name(w898) -> ("source"=w899:string)
              n334 = Format Into String(format string=w899, w897, w896) -> (resulting string=w900:string)  [unwired: 2 in, 1 out]
              n335 = Bundle By Name(cluster=w898, "source"=w900) -> (w895:errorcluster)
            }
            frame 1 {
              n336 = Initialize Array(w909) -> (w906:string[])  [unwired: 1 in]
              n337 = Unflatten From JSON(JSON string=w907, type and defaults=w906, error in (no error)=w908) -> (value=w905:string[], error out=w903:errorcluster)  [unwired: 4 in]
              n338 = String To Path(string=w905) -> (path=w902:path[])
              n339 = To Variant(anything=w902) -> (Variant=w904:variant)
            }
            frame 2 {
              n340 = Initialize Array(w917) -> (w914:string[][])  [unwired: 2 in]
              n341 = Unflatten From JSON(JSON string=w915, type and defaults=w914, error in (no error)=w916) -> (value=w913:string[][], error out=w911:errorcluster)  [unwired: 4 in]
              n342 = String To Path(string=w913) -> (path=w910:path[][])
              n343 = To Variant(anything=w910) -> (Variant=w912:variant)
            }
            frame 3 {
              n344 = Initialize Array(w925) -> (w922:string[][][])  [unwired: 3 in]
              n345 = Unflatten From JSON(JSON string=w923, type and defaults=w922, error in (no error)=w924) -> (value=w921:string[][][], error out=w919:errorcluster)  [unwired: 4 in]
              n346 = String To Path(string=w921) -> (path=w918:path[][][])
              n347 = To Variant(anything=w918) -> (Variant=w920:variant)
            }
            frame 4 {
              n348 = Initialize Array(w933) -> (w930:string[][][][])  [unwired: 4 in]
              n349 = Unflatten From JSON(JSON string=w931, type and defaults=w930, error in (no error)=w932) -> (value=w929:string[][][][], error out=w927:errorcluster)  [unwired: 4 in]
              n350 = String To Path(string=w929) -> (path=w926:path[][][][])
              n351 = To Variant(anything=w926) -> (Variant=w928:variant)
            }
          }
        }
        frame "Picture" {
          n352 = case shown="1" w941 {
            selector: w941 -> [w944 _ _ _ _]
            tunnel: "" -> [_ w957 w970 w987 w1008]
            tunnel: w939 -> [_ w956 w969 w986 w1007]
            tunnel: w938 -> [_ w955 w968 w985 w1006]
            tunnel: [w948 w953 w966 w983 w1004] -> w937
            tunnel: [w942 w951 w964 w981 w1002] -> w936
            tunnel: w935 -> [w948 _ _ _ _]
            tunnel: w934 -> [w943 _ _ _ _]
            frame Default {
              w945 = errorcluster {"status"=TRUE, "code"=1, "source"="%n-d Array of %s not handled."} ("error out")
              n353 = Unbundle By Name(w945) -> ("source"=w946:string)
              n354 = Format Into String(format string=w946, w944, w943) -> (resulting string=w947:string)  [unwired: 2 in, 1 out]
              n355 = Bundle By Name(cluster=w945, "source"=w947) -> (w942:errorcluster)
            }
            frame 1 {
              n356 = Initialize Array(w957) -> (w954:string[])  [unwired: 1 in]
              n357 = Unflatten From JSON(JSON string=w955, type and defaults=w954, error in (no error)=w956) -> (value=w950:string[], error out=w952:errorcluster)  [unwired: 4 in]
              n358 = for {
                shift-right: [w960] -> w951
                shift-left: w952 -> [w961]
                tunnel: w950 -> [w959] mode=indexing
                tunnel: [w958] -> w949 mode=indexing
                n359 = call <vilib>:"PNG Data to LV Image.vi"("error in (no error)"=w961, "png data"=w959) -> ("error out"=w960:errorcluster, "image data"=w958:T2)  [unwired: 8 in]
              }
              n360 = To Variant(anything=w949) -> (Variant=w953:variant)
            }
            frame 2 {
              n361 = Initialize Array(w970) -> (w967:string[][])  [unwired: 2 in]
              n362 = Unflatten From JSON(JSON string=w968, type and defaults=w967, error in (no error)=w969) -> (value=w963:string[][], error out=w965:errorcluster)  [unwired: 4 in]
              n363 = for {
                tunnel: w963 -> [w972] mode=indexing
                tunnel: [w971] -> w962
                shift-right: [w973] -> w964
                shift-left: w965 -> [w974]
                n364 = for {
                  shift-right: [w977] -> w973
                  shift-left: w974 -> [w978]
                  tunnel: w972 -> [w976] mode=indexing
                  tunnel: [w975] -> w971 mode=indexing
                  n365 = call <vilib>:"PNG Data to LV Image.vi"("error in (no error)"=w978, "png data"=w976) -> ("error out"=w977:errorcluster, "image data"=w975:T2)  [unwired: 8 in]
                }
              }
              n366 = To Variant(anything=w962) -> (Variant=w966:variant)
            }
            frame 3 {
              n367 = Initialize Array(w987) -> (w984:string[][][])  [unwired: 3 in]
              n368 = Unflatten From JSON(JSON string=w985, type and defaults=w984, error in (no error)=w986) -> (value=w980:string[][][], error out=w982:errorcluster)  [unwired: 4 in]
              n369 = for {
                tunnel: w980 -> [w989] mode=indexing
                tunnel: [w988] -> w979
                shift-right: [w990] -> w981
                shift-left: w982 -> [w991]
                n370 = for {
                  tunnel: w989 -> [w993] mode=indexing
                  tunnel: [w992] -> w988
                  shift-right: [w994] -> w990
                  shift-left: w991 -> [w995]
                  n371 = for {
                    shift-right: [w998] -> w994
                    shift-left: w995 -> [w999]
                    tunnel: w993 -> [w997] mode=indexing
                    tunnel: [w996] -> w992 mode=indexing
                    n372 = call <vilib>:"PNG Data to LV Image.vi"("error in (no error)"=w999, "png data"=w997) -> ("error out"=w998:errorcluster, "image data"=w996:T2)  [unwired: 8 in]
                  }
                }
              }
              n373 = To Variant(anything=w979) -> (Variant=w983:variant)
            }
            frame 4 {
              n374 = Initialize Array(w1008) -> (w1005:string[][][][])  [unwired: 4 in]
              n375 = Unflatten From JSON(JSON string=w1006, type and defaults=w1005, error in (no error)=w1007) -> (value=w1001:string[][][][], error out=w1003:errorcluster)  [unwired: 4 in]
              n376 = for {
                tunnel: w1001 -> [w1010] mode=indexing
                tunnel: [w1009] -> w1000
                shift-right: [w1011] -> w1002
                shift-left: w1003 -> [w1012]
                n377 = for {
                  tunnel: w1010 -> [w1014] mode=indexing
                  tunnel: [w1013] -> w1009
                  shift-right: [w1015] -> w1011
                  shift-left: w1012 -> [w1016]
                  n378 = for {
                    tunnel: w1014 -> [w1018] mode=indexing
                    tunnel: [w1017] -> w1013
                    shift-right: [w1019] -> w1015
                    shift-left: w1016 -> [w1020]
                    n379 = for {
                      shift-right: [w1023] -> w1019
                      shift-left: w1020 -> [w1024]
                      tunnel: w1018 -> [w1022] mode=indexing
                      tunnel: [w1021] -> w1017 mode=indexing
                      n380 = call <vilib>:"PNG Data to LV Image.vi"("error in (no error)"=w1024, "png data"=w1022) -> ("error out"=w1023:errorcluster, "image data"=w1021:T2)  [unwired: 8 in]
                    }
                  }
                }
              }
              n381 = To Variant(anything=w1000) -> (Variant=w1004:variant)
            }
          }
        }
        frame "Enum U8" {
          n382 = case shown="1" w1032 {
            selector: w1032 -> [w1035 _ _ _]
            tunnel: "" -> [_ w1051 w1066 w1084]
            tunnel: w1030 -> [_ w1050 w1065 w1083]
            tunnel: w1029 -> [_ w1049 w1064 w1082]
            tunnel: [w1039 w1047 w1062 w1080] -> w1028
            tunnel: [w1033 w1045 w1060 w1078] -> w1027
            tunnel: w1026 -> [w1039 w1040 w1055 w1073]
            tunnel: w1025 -> [w1034 _ _ _]
            frame Default {
              w1036 = errorcluster {"status"=TRUE, "code"=1, "source"="%n-d Array of %s not handled."} ("error out")
              n383 = Unbundle By Name(w1036) -> ("source"=w1037:string)
              n384 = Format Into String(format string=w1037, w1035, w1034) -> (resulting string=w1038:string)  [unwired: 2 in, 1 out]
              n385 = Bundle By Name(cluster=w1036, "source"=w1038) -> (w1033:errorcluster)
            }
            frame 1 {
              n386 = Initialize Array(w1051) -> (w1048:string[])  [unwired: 1 in]
              n387 = Unflatten From JSON(JSON string=w1049, type and defaults=w1048, error in (no error)=w1050) -> (value=w1044:string[], error out=w1046:errorcluster)  [unwired: 4 in]
              n388 = call <vilib>:"Get Numeric Information.vi"("error in (no error)"=w1046, "variant"=w1040) -> ("error out"=w1045:errorcluster, "enum names"=w1043:string[])  [unwired: 6 in, 2 out]
              n389 = for {
                tunnel: w1044 -> [w1053] mode=indexing
                tunnel: w1043 -> [w1054]
                tunnel: [w1052] -> w1042 mode=indexing
                n390 = Search 1D Array(1D array=w1054, element=w1053) -> (index of element=w1052:i32)  [unwired: 1 in]
              }
              n391 = To Unsigned Byte Integer(number=w1042) -> (unsigned 8bit integer=w1041:u8[])
              n392 = To Variant(anything=w1041) -> (Variant=w1047:variant)
            }
            frame 2 {
              n393 = Initialize Array(w1066) -> (w1063:string[][])  [unwired: 2 in]
              n394 = Unflatten From JSON(JSON string=w1064, type and defaults=w1063, error in (no error)=w1065) -> (value=w1059:string[][], error out=w1061:errorcluster)  [unwired: 4 in]
              n395 = call <vilib>:"Get Numeric Information.vi"("error in (no error)"=w1061, "variant"=w1055) -> ("error out"=w1060:errorcluster, "enum names"=w1058:string[])  [unwired: 6 in, 2 out]
              n396 = for {
                tunnel: w1059 -> [w1068] mode=indexing
                tunnel: w1058 -> [w1069]
                tunnel: [w1067] -> w1057 mode=indexing
                n397 = for {
                  tunnel: w1069 -> [w1072]
                  tunnel: w1068 -> [w1071] mode=indexing
                  tunnel: [w1070] -> w1067
                  n398 = Search 1D Array(1D array=w1072, element=w1071) -> (index of element=w1070:i32)  [unwired: 1 in]
                }
              }
              n399 = To Unsigned Byte Integer(number=w1057) -> (unsigned 8bit integer=w1056:u8[])
              n400 = To Variant(anything=w1056) -> (Variant=w1062:variant)
            }
            frame 3 {
              n401 = Initialize Array(w1084) -> (w1081:string[][][])  [unwired: 3 in]
              n402 = Unflatten From JSON(JSON string=w1082, type and defaults=w1081, error in (no error)=w1083) -> (value=w1077:string[][][], error out=w1079:errorcluster)  [unwired: 4 in]
              n403 = call <vilib>:"Get Numeric Information.vi"("error in (no error)"=w1079, "variant"=w1073) -> ("error out"=w1078:errorcluster, "enum names"=w1076:string[])  [unwired: 6 in, 2 out]
              n404 = for {
                tunnel: w1077 -> [w1086] mode=indexing
                tunnel: w1076 -> [w1087]
                tunnel: [w1085] -> w1075 mode=indexing
                n405 = for {
                  tunnel: w1087 -> [w1090]
                  tunnel: w1086 -> [w1089] mode=indexing
                  tunnel: [w1088] -> w1085 mode=indexing
                  n406 = for {
                    tunnel: w1090 -> [w1093]
                    tunnel: w1089 -> [w1092] mode=indexing
                    tunnel: [w1091] -> w1088
                    n407 = Search 1D Array(1D array=w1093, element=w1092) -> (index of element=w1091:i32)  [unwired: 1 in]
                  }
                }
              }
              n408 = To Unsigned Byte Integer(number=w1075) -> (unsigned 8bit integer=w1074:u8[][])
              n409 = To Variant(anything=w1074) -> (Variant=w1080:variant)
            }
          }
        }
        frame "Enum U16" {
          n410 = case shown="1" w1101 {
            selector: w1101 -> [w1104 _ _ _]
            tunnel: "" -> [_ w1120 w1135 w1153]
            tunnel: w1099 -> [_ w1119 w1134 w1152]
            tunnel: w1098 -> [_ w1118 w1133 w1151]
            tunnel: [w1108 w1116 w1131 w1149] -> w1097
            tunnel: [w1102 w1114 w1129 w1147] -> w1096
            tunnel: w1095 -> [w1108 w1109 w1124 w1142]
            tunnel: w1094 -> [w1103 _ _ _]
            frame Default {
              w1105 = errorcluster {"status"=TRUE, "code"=1, "source"="%n-d Array of %s not handled."} ("error out")
              n411 = Unbundle By Name(w1105) -> ("source"=w1106:string)
              n412 = Format Into String(format string=w1106, w1104, w1103) -> (resulting string=w1107:string)  [unwired: 2 in, 1 out]
              n413 = Bundle By Name(cluster=w1105, "source"=w1107) -> (w1102:errorcluster)
            }
            frame 1 {
              n414 = Initialize Array(w1120) -> (w1117:string[])  [unwired: 1 in]
              n415 = Unflatten From JSON(JSON string=w1118, type and defaults=w1117, error in (no error)=w1119) -> (value=w1113:string[], error out=w1115:errorcluster)  [unwired: 4 in]
              n416 = call <vilib>:"Get Numeric Information.vi"("error in (no error)"=w1115, "variant"=w1109) -> ("error out"=w1114:errorcluster, "enum names"=w1112:string[])  [unwired: 6 in, 2 out]
              n417 = for {
                tunnel: w1113 -> [w1122] mode=indexing
                tunnel: w1112 -> [w1123]
                tunnel: [w1121] -> w1111 mode=indexing
                n418 = Search 1D Array(1D array=w1123, element=w1122) -> (index of element=w1121:i32)  [unwired: 1 in]
              }
              n419 = To Unsigned Word Integer(number=w1111) -> (unsigned 16bit integer=w1110:u16[])
              n420 = To Variant(anything=w1110) -> (Variant=w1116:variant)
            }
            frame 2 {
              n421 = Initialize Array(w1135) -> (w1132:string[][])  [unwired: 2 in]
              n422 = Unflatten From JSON(JSON string=w1133, type and defaults=w1132, error in (no error)=w1134) -> (value=w1128:string[][], error out=w1130:errorcluster)  [unwired: 4 in]
              n423 = call <vilib>:"Get Numeric Information.vi"("error in (no error)"=w1130, "variant"=w1124) -> ("error out"=w1129:errorcluster, "enum names"=w1127:string[])  [unwired: 6 in, 2 out]
              n424 = for {
                tunnel: w1128 -> [w1137] mode=indexing
                tunnel: w1127 -> [w1138]
                tunnel: [w1136] -> w1126 mode=indexing
                n425 = for {
                  tunnel: w1138 -> [w1141]
                  tunnel: w1137 -> [w1140] mode=indexing
                  tunnel: [w1139] -> w1136
                  n426 = Search 1D Array(1D array=w1141, element=w1140) -> (index of element=w1139:i32)  [unwired: 1 in]
                }
              }
              n427 = To Unsigned Word Integer(number=w1126) -> (unsigned 16bit integer=w1125:u16[])
              n428 = To Variant(anything=w1125) -> (Variant=w1131:variant)
            }
            frame 3 {
              n429 = Initialize Array(w1153) -> (w1150:string[][][])  [unwired: 3 in]
              n430 = Unflatten From JSON(JSON string=w1151, type and defaults=w1150, error in (no error)=w1152) -> (value=w1146:string[][][], error out=w1148:errorcluster)  [unwired: 4 in]
              n431 = call <vilib>:"Get Numeric Information.vi"("error in (no error)"=w1148, "variant"=w1142) -> ("error out"=w1147:errorcluster, "enum names"=w1145:string[])  [unwired: 6 in, 2 out]
              n432 = for {
                tunnel: w1146 -> [w1155] mode=indexing
                tunnel: w1145 -> [w1156]
                tunnel: [w1154] -> w1144 mode=indexing
                n433 = for {
                  tunnel: w1156 -> [w1159]
                  tunnel: w1155 -> [w1158] mode=indexing
                  tunnel: [w1157] -> w1154 mode=indexing
                  n434 = for {
                    tunnel: w1159 -> [w1162]
                    tunnel: w1158 -> [w1161] mode=indexing
                    tunnel: [w1160] -> w1157
                    n435 = Search 1D Array(1D array=w1162, element=w1161) -> (index of element=w1160:i32)  [unwired: 1 in]
                  }
                }
              }
              n436 = To Unsigned Word Integer(number=w1144) -> (unsigned 16bit integer=w1143:u16[][])
              n437 = To Variant(anything=w1143) -> (Variant=w1149:variant)
            }
          }
        }
        frame "Enum U32" {
          n438 = case shown="2" w1170 {
            selector: w1170 -> [w1173 _ _ _]
            tunnel: "" -> [_ w1189 w1204 w1222]
            tunnel: w1168 -> [_ w1188 w1203 w1221]
            tunnel: w1167 -> [_ w1187 w1202 w1220]
            tunnel: [w1177 w1185 w1200 w1218] -> w1166
            tunnel: [w1171 w1183 w1198 w1216] -> w1165
            tunnel: w1164 -> [w1177 w1178 w1193 w1211]
            tunnel: w1163 -> [w1172 _ _ _]
            frame Default {
              w1174 = errorcluster {"status"=TRUE, "code"=1, "source"="%n-d Array of %s not handled."} ("error out")
              n439 = Unbundle By Name(w1174) -> ("source"=w1175:string)
              n440 = Format Into String(format string=w1175, w1173, w1172) -> (resulting string=w1176:string)  [unwired: 2 in, 1 out]
              n441 = Bundle By Name(cluster=w1174, "source"=w1176) -> (w1171:errorcluster)
            }
            frame 1 {
              n442 = Initialize Array(w1189) -> (w1186:string[])  [unwired: 1 in]
              n443 = Unflatten From JSON(JSON string=w1187, type and defaults=w1186, error in (no error)=w1188) -> (value=w1182:string[], error out=w1184:errorcluster)  [unwired: 4 in]
              n444 = call <vilib>:"Get Numeric Information.vi"("error in (no error)"=w1184, "variant"=w1178) -> ("error out"=w1183:errorcluster, "enum names"=w1181:string[])  [unwired: 6 in, 2 out]
              n445 = for {
                tunnel: w1182 -> [w1191] mode=indexing
                tunnel: w1181 -> [w1192]
                tunnel: [w1190] -> w1180 mode=indexing
                n446 = Search 1D Array(1D array=w1192, element=w1191) -> (index of element=w1190:i32)  [unwired: 1 in]
              }
              n447 = To Unsigned Long Integer(number=w1180) -> (unsigned 32bit integer=w1179:u32[])
              n448 = To Variant(anything=w1179) -> (Variant=w1185:variant)
            }
            frame 2 {
              n449 = Initialize Array(w1204) -> (w1201:string[][])  [unwired: 2 in]
              n450 = Unflatten From JSON(JSON string=w1202, type and defaults=w1201, error in (no error)=w1203) -> (value=w1197:string[][], error out=w1199:errorcluster)  [unwired: 4 in]
              n451 = call <vilib>:"Get Numeric Information.vi"("error in (no error)"=w1199, "variant"=w1193) -> ("error out"=w1198:errorcluster, "enum names"=w1196:string[])  [unwired: 6 in, 2 out]
              n452 = for {
                tunnel: w1197 -> [w1206] mode=indexing
                tunnel: w1196 -> [w1207]
                tunnel: [w1205] -> w1195 mode=indexing
                n453 = for {
                  tunnel: w1207 -> [w1210]
                  tunnel: w1206 -> [w1209] mode=indexing
                  tunnel: [w1208] -> w1205
                  n454 = Search 1D Array(1D array=w1210, element=w1209) -> (index of element=w1208:i32)  [unwired: 1 in]
                }
              }
              n455 = To Unsigned Long Integer(number=w1195) -> (unsigned 32bit integer=w1194:u32[])
              n456 = To Variant(anything=w1194) -> (Variant=w1200:variant)
            }
            frame 3 {
              n457 = Initialize Array(w1222) -> (w1219:string[][][])  [unwired: 3 in]
              n458 = Unflatten From JSON(JSON string=w1220, type and defaults=w1219, error in (no error)=w1221) -> (value=w1215:string[][][], error out=w1217:errorcluster)  [unwired: 4 in]
              n459 = call <vilib>:"Get Numeric Information.vi"("error in (no error)"=w1217, "variant"=w1211) -> ("error out"=w1216:errorcluster, "enum names"=w1214:string[])  [unwired: 6 in, 2 out]
              n460 = for {
                tunnel: w1215 -> [w1224] mode=indexing
                tunnel: w1214 -> [w1225]
                tunnel: [w1223] -> w1213 mode=indexing
                n461 = for {
                  tunnel: w1225 -> [w1228]
                  tunnel: w1224 -> [w1227] mode=indexing
                  tunnel: [w1226] -> w1223 mode=indexing
                  n462 = for {
                    tunnel: w1228 -> [w1231]
                    tunnel: w1227 -> [w1230] mode=indexing
                    tunnel: [w1229] -> w1226
                    n463 = Search 1D Array(1D array=w1231, element=w1230) -> (index of element=w1229:i32)  [unwired: 1 in]
                  }
                }
              }
              n464 = To Unsigned Long Integer(number=w1213) -> (unsigned 32bit integer=w1212:u32[][])
              n465 = To Variant(anything=w1212) -> (Variant=w1218:variant)
            }
          }
        }
        frame "Enum U64" {
          n466 = case shown="1" w1239 {
            selector: w1239 -> [w1242 _ _ _]
            tunnel: "" -> [_ w1258 w1273 w1291]
            tunnel: w1237 -> [_ w1257 w1272 w1290]
            tunnel: w1236 -> [_ w1256 w1271 w1289]
            tunnel: [w1246 w1254 w1269 w1287] -> w1235
            tunnel: [w1240 w1252 w1267 w1285] -> w1234
            tunnel: w1233 -> [w1246 w1247 w1262 w1280]
            tunnel: w1232 -> [w1241 _ _ _]
            frame Default {
              w1243 = errorcluster {"status"=TRUE, "code"=1, "source"="%n-d Array of %s not handled."} ("error out")
              n467 = Unbundle By Name(w1243) -> ("source"=w1244:string)
              n468 = Format Into String(format string=w1244, w1242, w1241) -> (resulting string=w1245:string)  [unwired: 2 in, 1 out]
              n469 = Bundle By Name(cluster=w1243, "source"=w1245) -> (w1240:errorcluster)
            }
            frame 1 {
              n470 = Initialize Array(w1258) -> (w1255:string[])  [unwired: 1 in]
              n471 = Unflatten From JSON(JSON string=w1256, type and defaults=w1255, error in (no error)=w1257) -> (value=w1251:string[], error out=w1253:errorcluster)  [unwired: 4 in]
              n472 = call <vilib>:"Get Numeric Information.vi"("error in (no error)"=w1253, "variant"=w1247) -> ("error out"=w1252:errorcluster, "enum names"=w1250:string[])  [unwired: 6 in, 2 out]
              n473 = for {
                tunnel: w1251 -> [w1260] mode=indexing
                tunnel: w1250 -> [w1261]
                tunnel: [w1259] -> w1249 mode=indexing
                n474 = Search 1D Array(1D array=w1261, element=w1260) -> (index of element=w1259:i32)  [unwired: 1 in]
              }
              n475 = To Unsigned Quad Integer(1:w1249) -> (0:w1248:u64[])
              n476 = To Variant(anything=w1248) -> (Variant=w1254:variant)
            }
            frame 2 {
              n477 = Initialize Array(w1273) -> (w1270:string[][])  [unwired: 2 in]
              n478 = Unflatten From JSON(JSON string=w1271, type and defaults=w1270, error in (no error)=w1272) -> (value=w1266:string[][], error out=w1268:errorcluster)  [unwired: 4 in]
              n479 = call <vilib>:"Get Numeric Information.vi"("error in (no error)"=w1268, "variant"=w1262) -> ("error out"=w1267:errorcluster, "enum names"=w1265:string[])  [unwired: 6 in, 2 out]
              n480 = for {
                tunnel: w1266 -> [w1275] mode=indexing
                tunnel: w1265 -> [w1276]
                tunnel: [w1274] -> w1264 mode=indexing
                n481 = for {
                  tunnel: w1276 -> [w1279]
                  tunnel: w1275 -> [w1278] mode=indexing
                  tunnel: [w1277] -> w1274
                  n482 = Search 1D Array(1D array=w1279, element=w1278) -> (index of element=w1277:i32)  [unwired: 1 in]
                }
              }
              n483 = To Unsigned Quad Integer(1:w1264) -> (0:w1263:u64[])
              n484 = To Variant(anything=w1263) -> (Variant=w1269:variant)
            }
            frame 3 {
              n485 = Initialize Array(w1291) -> (w1288:string[][][])  [unwired: 3 in]
              n486 = Unflatten From JSON(JSON string=w1289, type and defaults=w1288, error in (no error)=w1290) -> (value=w1284:string[][][], error out=w1286:errorcluster)  [unwired: 4 in]
              n487 = call <vilib>:"Get Numeric Information.vi"("error in (no error)"=w1286, "variant"=w1280) -> ("error out"=w1285:errorcluster, "enum names"=w1283:string[])  [unwired: 6 in, 2 out]
              n488 = for {
                tunnel: w1284 -> [w1293] mode=indexing
                tunnel: w1283 -> [w1294]
                tunnel: [w1292] -> w1282 mode=indexing
                n489 = for {
                  tunnel: w1294 -> [w1297]
                  tunnel: w1293 -> [w1296] mode=indexing
                  tunnel: [w1295] -> w1292 mode=indexing
                  n490 = for {
                    tunnel: w1297 -> [w1300]
                    tunnel: w1296 -> [w1299] mode=indexing
                    tunnel: [w1298] -> w1295
                    n491 = Search 1D Array(1D array=w1300, element=w1299) -> (index of element=w1298:i32)  [unwired: 1 in]
                  }
                }
              }
              n492 = To Unsigned Quad Integer(1:w1282) -> (0:w1281:u64[][])
              n493 = To Variant(anything=w1281) -> (Variant=w1287:variant)
            }
          }
        }
        frame Default {
          w1304 = errorcluster {"status"=TRUE, "code"=1, "source"="Addray data type '%s' no supported."} ("error out")
          n494 = Unbundle By Name(w1304) -> ("source"=w1305:string)
          n495 = Format Into String(format string=w1305, w1303) -> (resulting string=w1306:string)  [unwired: 2 in, 1 out]
          n496 = Bundle By Name(cluster=w1304, "source"=w1306) -> (w1302:errorcluster)
        }
      }
    }
    frame "Cluster" {
      n497 = call <vilib>:"Get Cluster Information.vi"("error in (no error)"=w1312, "variant"=w1308) -> ("error out"=w1310:errorcluster, "cluster elements"=w1311:variant[])  [unwired: 8 in]
      n498 = for {
        tunnel: w1311 -> [w1319] mode=indexing
        shift-right: [w1314] -> w1309
        shift-left: w1310 -> [w1323]
        tunnel: w1307 -> [w1321]
        n499 = call <vilib>:"Get Type Information.vi"("error in (no error)"=w1323, "variant"=w1319) -> ("error out"=w1322:errorcluster, "name"=w1313:string, "type"=w1317:T1)  [unwired: 5 in, 2 out]
        n500 = Build Array(w1313) -> (w1320:string[])
        n501 = Unflatten From JSON(path=w1320, JSON string=w1321, type and defaults="", error in (no error)=w1322) -> (value=w1316:string, error out=w1315:errorcluster)  [unwired: 3 in]
        n502 = case shown="Default" w1317 {
          tunnel: w1316 -> [_]
          tunnel: w1315 -> [_]
          tunnel: [w1325] -> w1314
          tunnel: w1313 -> [w1324]
          frame Default {
            w1326 = errorcluster {"status"=TRUE, "code"=1, "source"="Data type '%s' no supported."} ("error out")
            n503 = Unbundle By Name(w1326) -> ("source"=w1327:string)
            n504 = Format Into String(format string=w1327, w1324) -> (resulting string=w1328:string)  [unwired: 2 in, 1 out]
            n505 = Bundle By Name(cluster=w1326, "source"=w1328) -> (w1325:errorcluster)
          }
        }
      }
    }
    frame "I16" {
      n506 = Scan From String(input string=w1332, error in=w1334, default 1=i16 0 ("default value 1")) -> (error out=w1333:errorcluster, output 1=w1329:i16)  [unwired: 2 in, 2 out]
      n507 = To Variant(anything=w1329) -> (Variant=w1330:variant)
    }
    frame "I32" {
      n508 = Scan From String(input string=w1338, error in=w1340, default 1=0 ("default value 1")) -> (error out=w1339:errorcluster, output 1=w1335:i32)  [unwired: 2 in, 2 out]
      n509 = To Variant(anything=w1335) -> (Variant=w1336:variant)
    }
    frame "I64" {
      n510 = Scan From String(input string=w1344, error in=w1346, default 1=i64 0 ("default value 1")) -> (error out=w1345:errorcluster, output 1=w1341:i64)  [unwired: 2 in, 2 out]
      n511 = To Variant(anything=w1341) -> (Variant=w1342:variant)
    }
    frame "U8" {
      n512 = Scan From String(input string=w1350, error in=w1352, default 1=u8 0 ("default value 1")) -> (error out=w1351:errorcluster, output 1=w1347:u8)  [unwired: 2 in, 2 out]
      n513 = To Variant(anything=w1347) -> (Variant=w1348:variant)
    }
    frame "U16" {
      n514 = Scan From String(input string=w1356, error in=w1358, default 1=u16 0 ("default value 1")) -> (error out=w1357:errorcluster, output 1=w1353:u16)  [unwired: 2 in, 2 out]
      n515 = To Variant(anything=w1353) -> (Variant=w1354:variant)
    }
    frame "U32" {
      n516 = Scan From String(input string=w1362, error in=w1364, default 1=u32 0 ("default value 1")) -> (error out=w1363:errorcluster, output 1=w1359:u32)  [unwired: 2 in, 2 out]
      n517 = To Variant(anything=w1359) -> (Variant=w1360:variant)
    }
    frame "U64" {
      n518 = Scan From String(input string=w1368, error in=w1370, default 1=u64 0 ("default value 1")) -> (error out=w1369:errorcluster, output 1=w1365:u64)  [unwired: 2 in, 2 out]
      n519 = To Variant(anything=w1365) -> (Variant=w1366:variant)
    }
    frame "Single Float" {
      n520 = Scan From String(input string=w1374, error in=w1376, default 1=sgl 0.0 ("default value 1")) -> (error out=w1375:errorcluster, output 1=w1371:sgl)  [unwired: 2 in, 2 out]
      n521 = To Variant(anything=w1371) -> (Variant=w1372:variant)
    }
    frame "Single Float With Unit" {
      n522 = Scan From String(input string=w1380, error in=w1382, default 1=sgl 0.0 ("default value 1")) -> (error out=w1381:errorcluster, output 1=w1377:sgl)  [unwired: 2 in, 2 out]
      n523 = To Variant(anything=w1377) -> (Variant=w1378:variant)
    }
    frame "Double Float" {
      n524 = Scan From String(input string=w1386, error in=w1388, default 1=0.0 ("default value 1")) -> (error out=w1387:errorcluster, output 1=w1383:dbl)  [unwired: 2 in, 2 out]
      n525 = To Variant(anything=w1383) -> (Variant=w1384:variant)
    }
    frame "Double Float With Unit" {
      n526 = Scan From String(input string=w1392, error in=w1394, default 1=0.0 ("default value 1")) -> (error out=w1393:errorcluster, output 1=w1389:dbl)  [unwired: 2 in, 2 out]
      n527 = To Variant(anything=w1389) -> (Variant=w1390:variant)
    }
    frame "Extended Float" {
      n528 = Scan From String(input string=w1398, error in=w1400, default 1=ext 0.0 ("default value 1")) -> (error out=w1399:errorcluster, output 1=w1395:ext)  [unwired: 2 in, 2 out]
      n529 = To Variant(anything=w1395) -> (Variant=w1396:variant)
    }
    frame "Extended Float With Unit" {
      n530 = Scan From String(input string=w1404, error in=w1406, default 1=ext 0.0 ("default value 1")) -> (error out=w1405:errorcluster, output 1=w1401:ext)  [unwired: 2 in, 2 out]
      n531 = To Variant(anything=w1401) -> (Variant=w1402:variant)
    }
    frame "Single Complex" {
      n532 = Scan From String(input string=w1410, error in=w1412, default 1=csg 0.0+0.0i ("default value 1")) -> (error out=w1411:errorcluster, output 1=w1407:csg)  [unwired: 2 in, 2 out]
      n533 = To Variant(anything=w1407) -> (Variant=w1408:variant)
    }
    frame "Single Complex with Unit" {
      n534 = Scan From String(input string=w1416, error in=w1418, default 1=csg 0.0+0.0i ("default value 1")) -> (error out=w1417:errorcluster, output 1=w1413:csg)  [unwired: 2 in, 2 out]
      n535 = To Variant(anything=w1413) -> (Variant=w1414:variant)
    }
    frame "Double Complex" {
      n536 = Scan From String(input string=w1422, error in=w1424, default 1=cdb 0.0+0.0i ("default value 1")) -> (error out=w1423:errorcluster, output 1=w1419:cdb)  [unwired: 2 in, 2 out]
      n537 = To Variant(anything=w1419) -> (Variant=w1420:variant)
    }
    frame "Double Complex with Unit" {
      n538 = Scan From String(input string=w1428, error in=w1430, default 1=cdb 0.0+0.0i ("default value 1")) -> (error out=w1429:errorcluster, output 1=w1425:cdb)  [unwired: 2 in, 2 out]
      n539 = To Variant(anything=w1425) -> (Variant=w1426:variant)
    }
    frame "Extended Complex" {
      n540 = Scan From String(input string=w1434, error in=w1436, default 1=cxt 0.0+0.0i ("default value 1")) -> (error out=w1435:errorcluster, output 1=w1431:cxt)  [unwired: 2 in, 2 out]
      n541 = To Variant(anything=w1431) -> (Variant=w1432:variant)
    }
    frame "Extended Complex with Unit" {
      n542 = Scan From String(input string=w1440, error in=w1442, default 1=cxt 0.0+0.0i ("default value 1")) -> (error out=w1441:errorcluster, output 1=w1437:cxt)  [unwired: 2 in, 2 out]
      n543 = To Variant(anything=w1437) -> (Variant=w1438:variant)
    }
    frame "Enum U8" {
      n544 = call <vilib>:"Get Numeric Information.vi"("error in (no error)"=w1448, "variant"=w1449) -> ("error out"=w1444:errorcluster, "enum names"=w1447:string[])  [unwired: 6 in, 2 out]
      n545 = Search 1D Array(1D array=w1447, element=w1446) -> (index of element=w1445:i32)  [unwired: 1 in]
      n546 = To Unsigned Byte Integer(number=w1445) -> (unsigned 8bit integer=w1443:u8)
      n547 = To Variant(anything=w1443) -> (Variant=w1450:variant)
    }
    frame "Enum U16" {
      n548 = call <vilib>:"Get Numeric Information.vi"("error in (no error)"=w1456, "variant"=w1457) -> ("error out"=w1452:errorcluster, "enum names"=w1455:string[])  [unwired: 6 in, 2 out]
      n549 = Search 1D Array(1D array=w1455, element=w1454) -> (index of element=w1453:i32)  [unwired: 1 in]
      n550 = To Unsigned Word Integer(number=w1453) -> (unsigned 16bit integer=w1451:u16)
      n551 = To Variant(anything=w1451) -> (Variant=w1458:variant)
    }
    frame "Enum U32" {
      n552 = call <vilib>:"Get Numeric Information.vi"("error in (no error)"=w1464, "variant"=w1465) -> ("error out"=w1460:errorcluster, "enum names"=w1463:string[])  [unwired: 6 in, 2 out]
      n553 = Search 1D Array(1D array=w1463, element=w1462) -> (index of element=w1461:i32)  [unwired: 1 in]
      n554 = To Unsigned Long Integer(number=w1461) -> (unsigned 32bit integer=w1459:u32)
      n555 = To Variant(anything=w1459) -> (Variant=w1466:variant)
    }
    frame "Enum U64" {
      n556 = call <vilib>:"Get Numeric Information.vi"("error in (no error)"=w1472, "variant"=w1473) -> ("error out"=w1468:errorcluster, "enum names"=w1471:string[])  [unwired: 6 in, 2 out]
      n557 = Search 1D Array(1D array=w1471, element=w1470) -> (index of element=w1469:i32)  [unwired: 1 in]
      n558 = To Unsigned Quad Integer(1:w1469) -> (0:w1467:u64)
      n559 = To Variant(anything=w1467) -> (Variant=w1474:variant)
    }
    frame Default {
      w1476 = errorcluster {"status"=TRUE, "code"=1, "source"="Data type '%s' no supported."} ("error out")
      n560 = Unbundle By Name(w1476) -> ("source"=w1478:string)
      n561 = Format Into String(format string=w1478, w1477) -> (resulting string=w1479:string)  [unwired: 2 in, 1 out]
      n562 = Bundle By Name(cluster=w1476, "source"=w1479) -> (w1475:errorcluster)
    }
  }
  "error out" <- w6
  "Type/Default out" <- w4
